vi "hostCommander_dualVStim_beta.vi"() -> ()   [LabVIEW 2014]
uses:
  <vilib>/Platform/TimedLoop/XDataNode/timing_clust.ctl
  <vilib>/Platform/TimedLoop/XDataNode/nitl_modes.ctl
  <vilib>/Platform/TimedLoop/XDataNode/wakeup.ctl
  <vilib>/dex/Stream Element Allocation Mode.ctl
  <vilib>/platform/TimedLoop/XDataNode/XDataNode.xnode
  <resource>/objmgr/ni.dex.rc
  <vilib>/Platform/TimedLoop/XDataNode/XDNodeRunTimeDep.lvlib
  <vilib>/Analysis/NI_AALBase.lvlib
  <vilib>/Analysis/1siggen.llb/Riffle Array (I32).vi
panel:
  in  "allowCorrection 2":bool
  out "Tab Control":enum32{"Host Commander"}(tab)
  out "rightReward":dbl format="%.2f"
  out "leftReward":dbl format="%.2f"
  out "rightLick":dbl format="%.2f"
  out "leftLick":dbl format="%.2f"
  out "reward#":i32=500
  in  "tickRate":u32=1
  in  "displayLength":dbl=10.0
  out "CurTrial#":u16
  out "Digital Waveform Graph":digitalwaveform(graph)
  out "stateMissed":bool
  out "VSmissed":bool
  out "VSbusy":bool=TRUE caption="VS"
  out "stateBusy":bool=TRUE caption="State"
  in  "FileName":string="debug"
  in  "Save data":bool=TRUE
  in  "Tab Control _2":T1(tab)
  in  "trialKey":i32[](array[numeric])
  in  "left":dbl=0.5 format="%.2f"
  in  "right":dbl=0.5 format="%.2f"
  in  "Initializeation Screen":dbl
  in  "Repeat":dbl
  in  "Interleave":bool
  in  "Randominze":bool
  in  "Blank":bool
  in  "Timing":sgl[](array[numeric])=[0.1, 0.2, 0.4, 0.6, 0.8, 1.0]
  in  "Orientation":sgl[](array[numeric])=[0.1, 0.2, 0.4, 0.6, 0.8, 1.0]
  in  "TF":sgl[](array[numeric])=[0.1, 0.2, 0.4, 0.6, 0.8, 1.0]
  in  "VS type":string(combo)="DelayedMatchToSampleMove"
  in  "SF":sgl[](array[numeric])=[0.04, 0.08, 0.16, 0.32, 0.45]
  in  "rtFIFOsize":u32=50
  in  "rtFIFOtimeout":u32
  in  "rtFIFOdataPool":u32=20
  in  "stateMachineCycle_uS":i64=500
  in  "minDelay":i32
  in  "maxDelay":i32=2000000
  in  "autoAllowCorrection":bool=TRUE
  in  "allowCorrection":bool
  in  "autoDelay":bool
  in  "vsFilterPeriod_uS":i32=500 format="%#1.6f"
  in  "lickThreshold_V":fxp<+/-,16,5>=1.0 format="%#.4f"
  in  "vsThreshold_V":fxp<+/-,16,5>=2.0 format="%#.4f"
  in  "audioThreshold_V":fxp<+/-,16,5>=2.2998046875 format="%.4f"
  in  "audioFilterPeriod_uS":i32=500 format="%#1.6f"
  in  "audioOffState_V":fxp<+/-,16,5> format="%#.4f"
  in  "manualShock":bool
  in  "manualWaterRight":bool
  in  "manualWaterLeft":bool
  in  "lickReward":bool
  in  "allowPunish":bool
  in  "beh type":string="LeftRight"
  in  "toneReward":bool
  in  "rwdrefPeriod_uS":u32=1000000
  in  "rewardPeriod_uS":u32=3000000
  in  "waterOn_uS":u32=35000
  in  "timeout_uS":u32=5000000
  in  "shockOn_uS":u32
  in  "delay_uS":u32=500000
  out "current state":u16(ring) items=["idle", "vs before", "vs", "vs after", "delay", "tone before", "tone", "tone after", "cycle end", "reward", "reward refractory", "punish", "punish refractory", "timeout", "exit"]
  out "case2":i32
  out "case1":i32
  in  "forceLeftTrial":bool
  in  "forceRightTrial":bool
  in  "forceCorrTrial":bool
  in  "autoCorrTrial":bool=TRUE
  in  "autoTimeout":bool
  in  "autoStop":bool
  in  "autoStopAtReward#":i32=250
  in  "updateEveryTrial#":u16=10
  in  "maxTimeout":i32=8000000
  out "newStartTrial#":i32
  out "newStartReward#":i32
  out "contNoRewardAccum":i32
  out "contNoReward":i32
  out "contReward":i32
  out "curPerformance":dbl format="%.2f"
  out "overallPerformance":dbl format="%.2f"
  in  "waterPunish":bool
  in  "No VS":bool
  out "Error 1":string
  out "Error 2":string
  out "Originating IP":string="192.168.137.2"
  out "Incoming data":string="TrlDone 1.000 "
  out "stream counter":u32
  out "Is Connected":bool
  out "Available Elements for Writing":i32
  in  "stream writer buffer size":i32=500
  in  "IP_VS":string="192.168.137.3"
  in  "IP_RT":string="192.168.137.2"
  in  "port_remote":u16=9091
  in  "IP_host":string="192.168.137.1"
  in  "port_local":u16=9090
  in  "IP_broadcast":string="192.168.137.255"
  out "INFO":string="Stop 1.000 "
  out "stop - local":bool=TRUE
  in  "Notes":string="14-4"
  in  "Abort":bool caption="run-stop"
  in  "run-stop":bool
  out "dispTimeout":bool
  out "saveTimeout":bool
  out "CurTrial# (remote)":u16
  in  "totalTrial#":u16=600
  out "CurTime":i32
  in  "ITI_ms":dbl=2000.0
  out "CurTime (sec)":i32
  in  "FilePath":string="D:\\BehData\\"
  # "busy"
  # "missed"
  # "min"
  # "sec"
  # "trialProbability"
  # "Errors for debugging"
types:
  T1 = enum32{"Visual Stimuli", "State Machine", "Behavior", "Network", "Notes"}
  T2 = enum16{"open", "replace", "create", "open or create", "replace or create", "replace or create with confirmation"}
  T3 = enum16{"big-endian, network order", "native, host order", "little-endian"}
  T4 = typedef "XDNodeRunTimeDep.lvlib/timing_clust.ctl" = cluster{"Expected End [f-1]":u64, "Actual End [f-1]":u64, "Finished Late? [f-1]":bool, "Expected End [i-1]":u64, "Actual End [i-1]":u64, "Finished Late? [i-1]":bool, "Expected Start [i]":u64, "Actual Start [i]":u64, "Expected Start [f]":u64, "Actual Start [f]":u64, "Source Name":string, "Structure Name":string, "Period":i64, "Deadline":i64, "Offset":i64, "Start":i64, "Priority":i32, "Timeout":i32, "Mode":T5, "Wakeup Reason":T6, "Error":errorcluster, "Source Type":string, "Secondary Source Type":string, "Global End Time":u64, "Global Start Time":u64, "Frame Duration":u64, "Iteration Duration":u64, "Assigned CPU":i32, "I/O Scan Engine Mode":u32}
  T5 = typedef "XDNodeRunTimeDep.lvlib/nitl_modes.ctl" = enum32{"No Change", "Process missed periods, maintain original phase", "Discard missed periods, maintain original phase", "Process missed periods, ignore original phase", "Discard missed periods, ignore original phase"}
  T6 = typedef "XDNodeRunTimeDep.lvlib/wakeup.ctl" = enum32{"Normal", "Aborted", "Asynchronous wakeup", "Timing source error", "Timed loop error", "Timeout"}
  T7 = typedef "Stream Element Allocation Mode.ctl" = u32
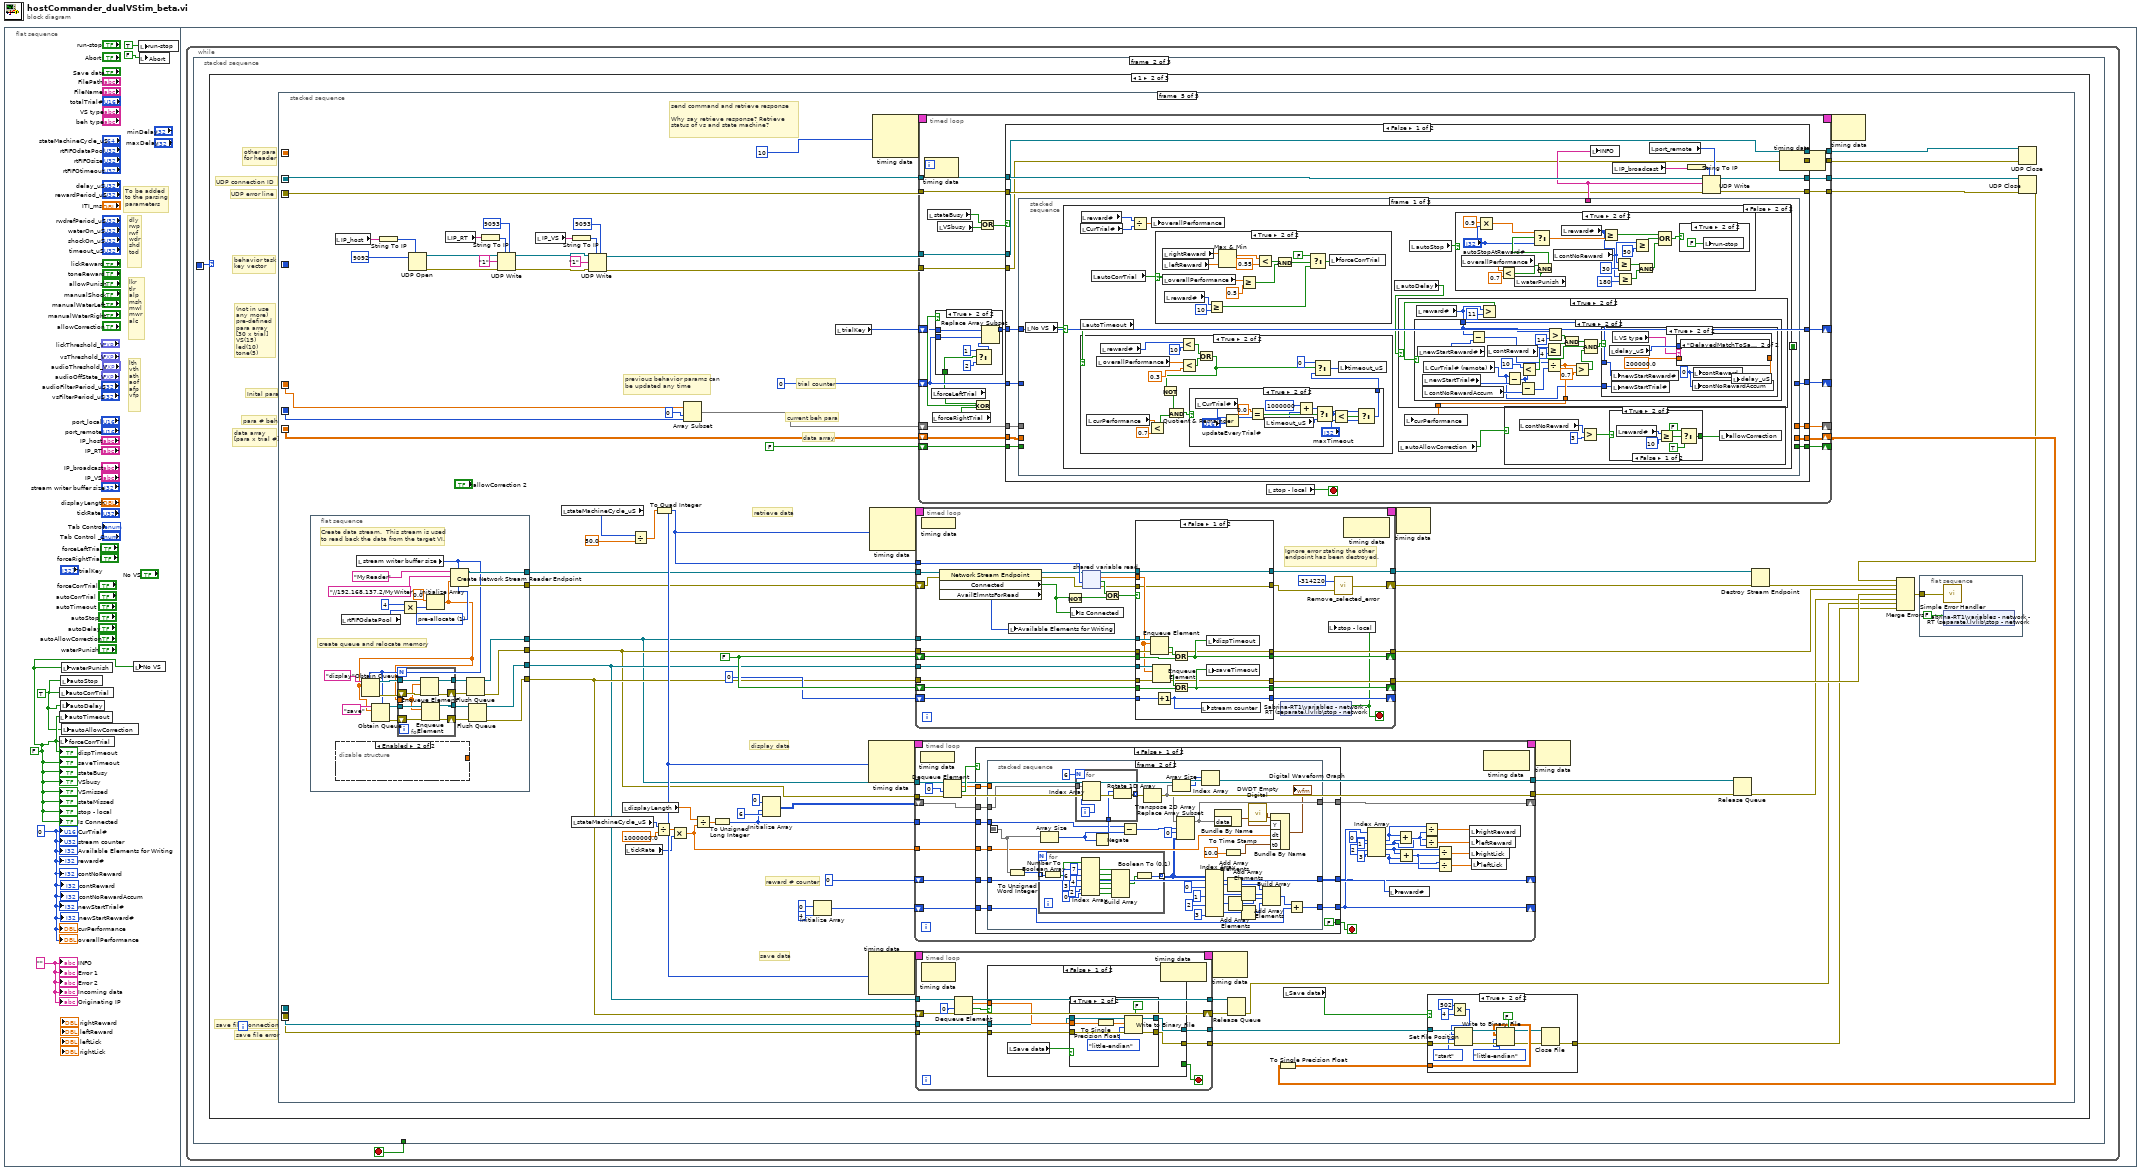
[diagram p0: block diagram]
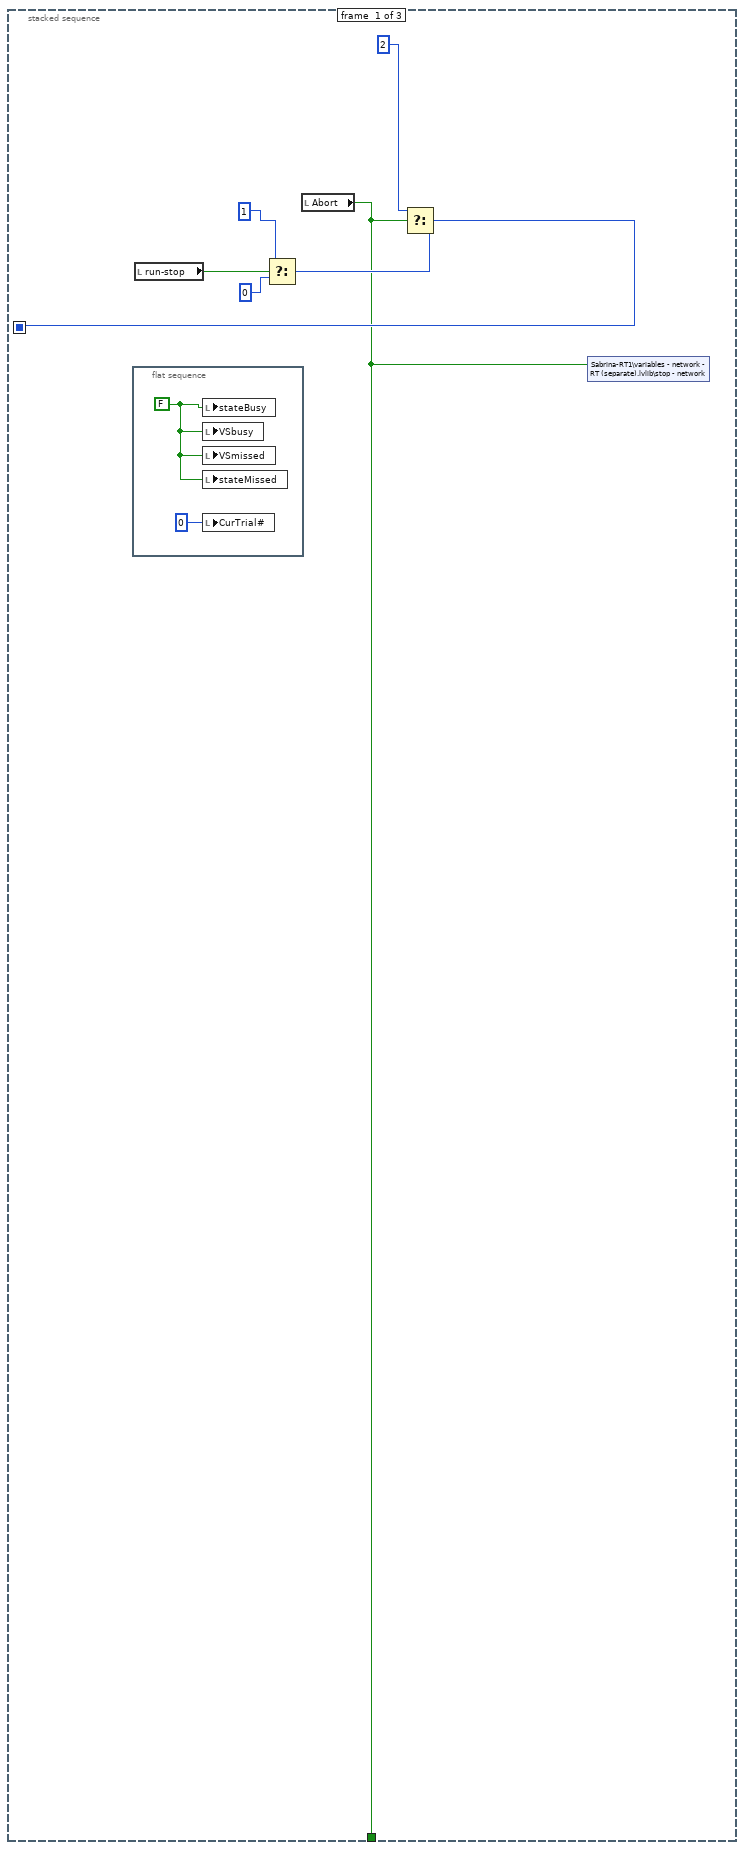
[diagram p2: hidden frame]
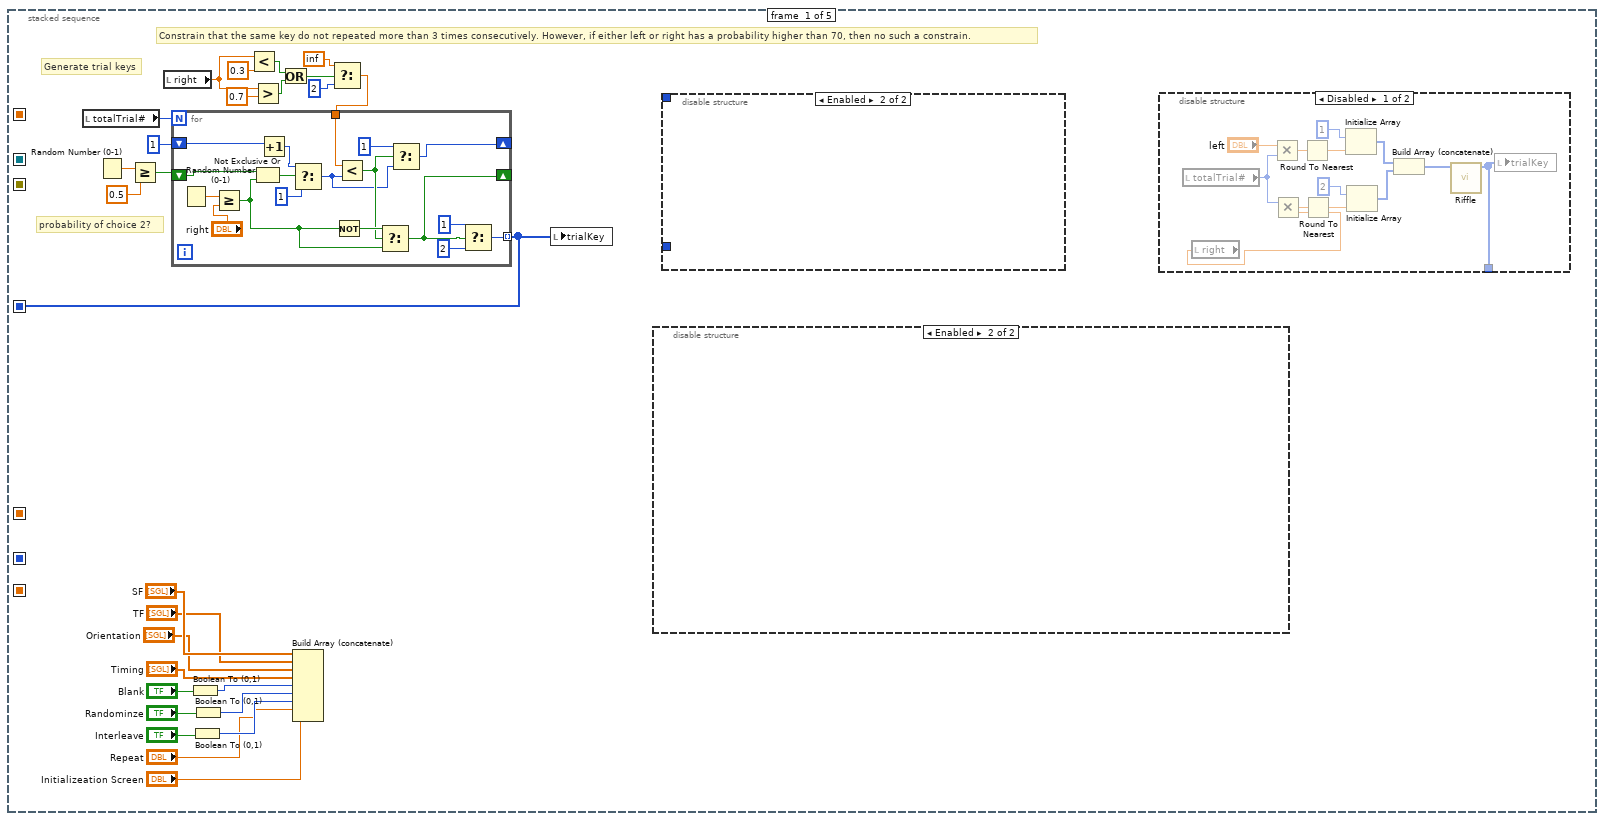
[diagram p4: hidden frame]
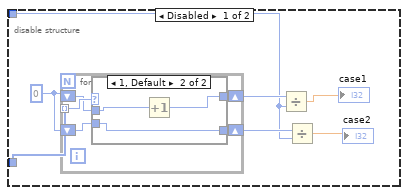
[diagram p5: hidden frame]
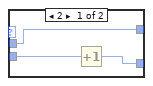
[diagram p6: hidden frame]
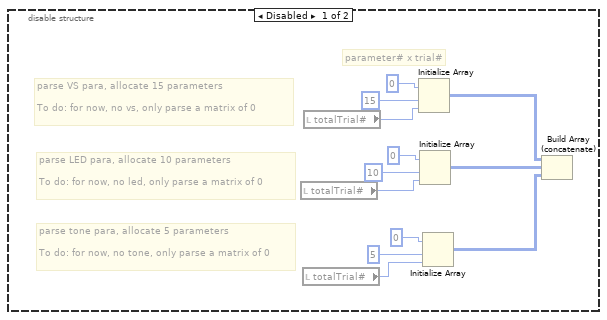
[diagram p8: hidden frame]
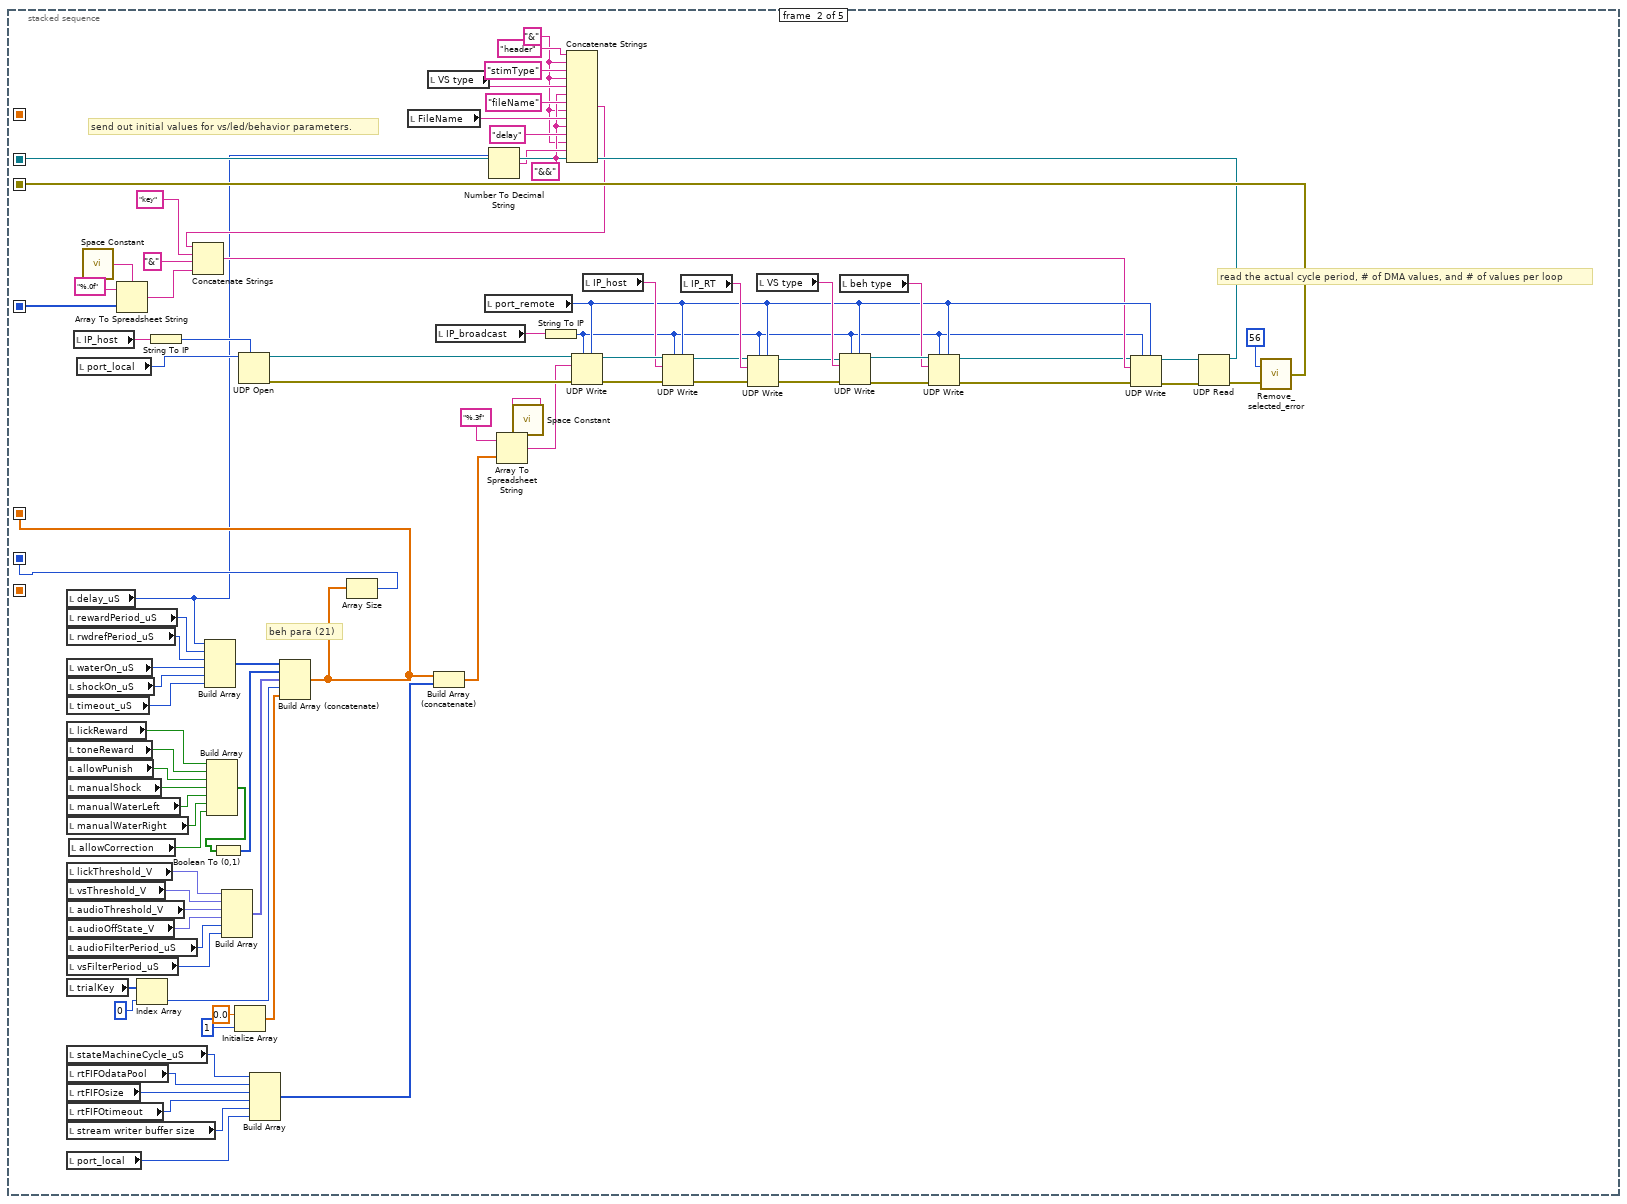
[diagram p9: hidden frame]
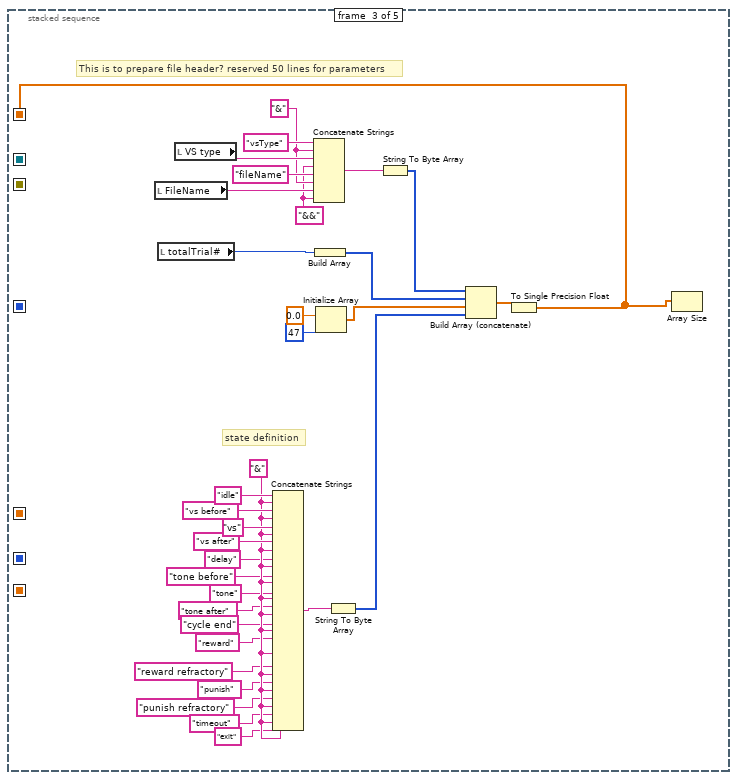
[diagram p10: hidden frame]
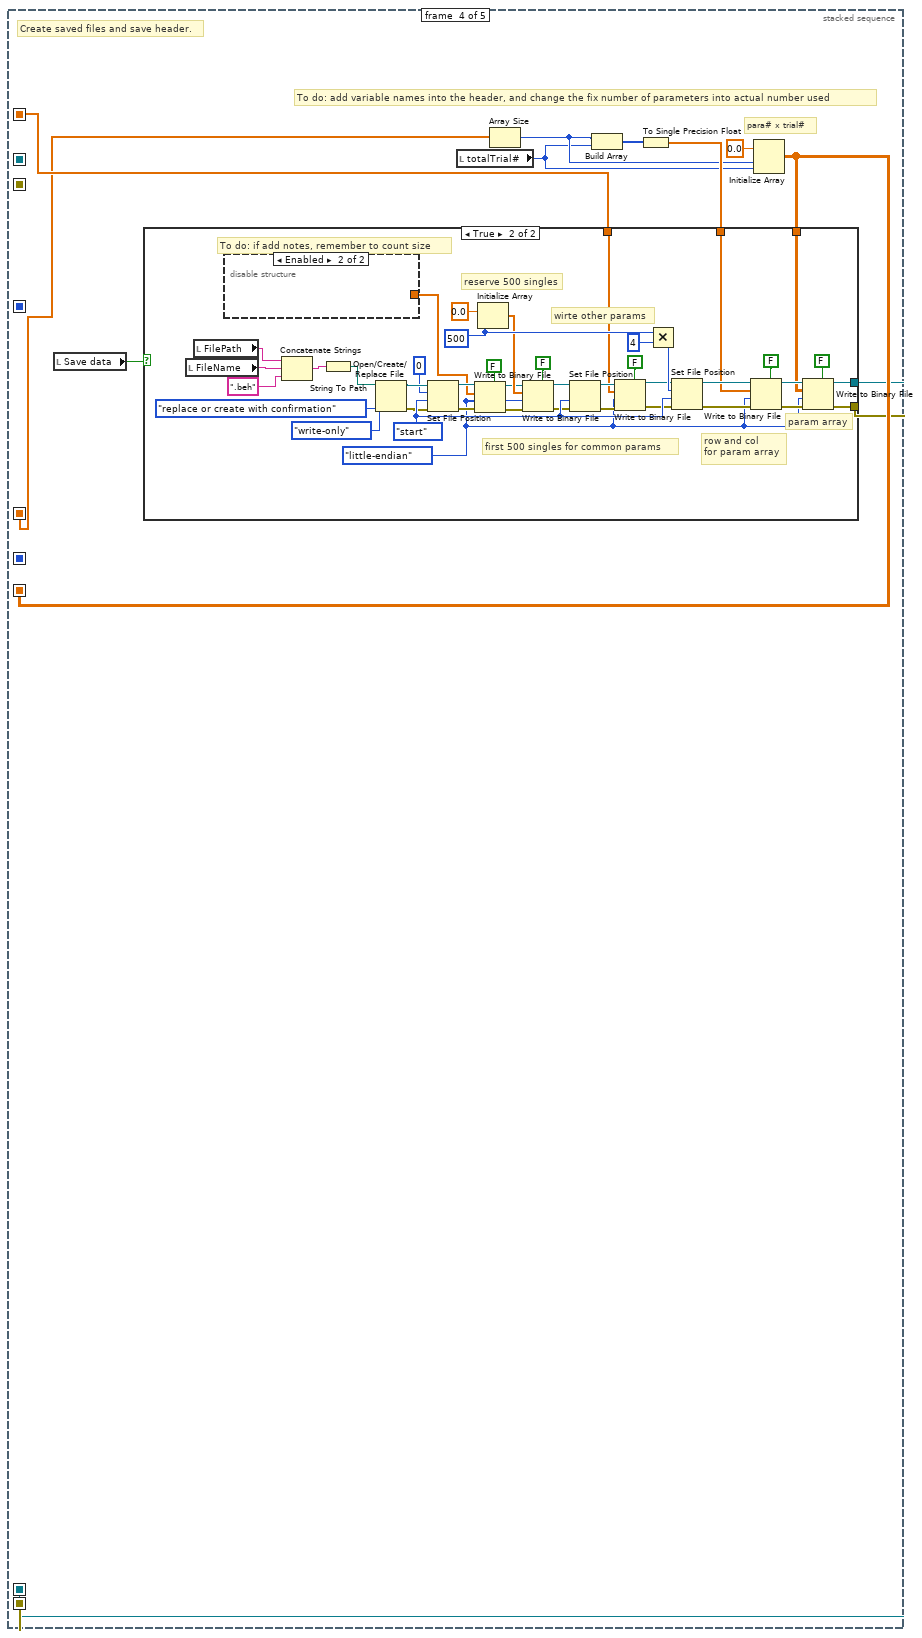
[diagram p11: hidden frame]
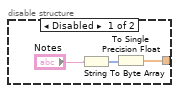
[diagram p13: hidden frame]
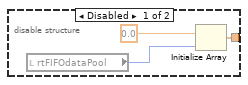
[diagram p14: hidden frame]
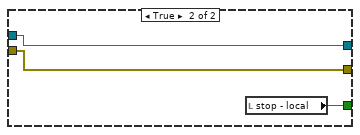
[diagram p16: hidden frame]
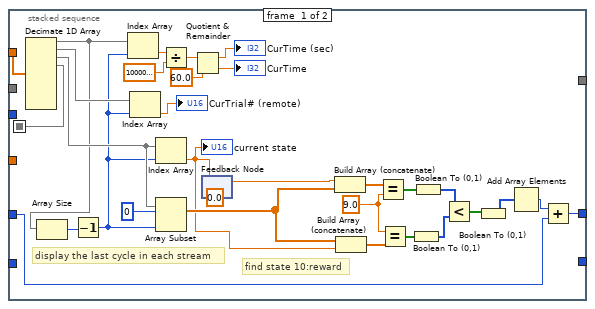
[diagram p17: hidden frame]
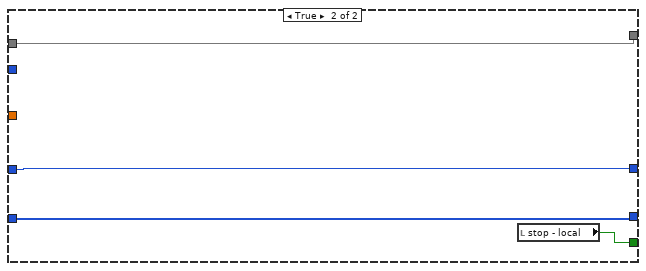
[diagram p18: hidden frame]
diagram:
  n1 = flat-sequence {
    frame #0 {
      w1 = TRUE
      w4 = ""
      w3 = 0
      w2 = FALSE
      # "To be added\nto the parsing\nparameters"
      # "lth\nvth\nath\naof\nafp\nvfp"
      # "dly\nrwp\nrwf\nwdr\nshd\ntod"
      # "lkr\ntlr\nalp\nmsh\nmwl\nmwr\nalc"
      n2 = local write "autoTimeout"(w2) -> ()
      n3 = local write "forceCorrTrial"(w2) -> ()
      n4 = local write "autoCorrTrial"(w1) -> ()
      n5 = local write "autoDelay"(w1) -> ()
      n6 = local write "autoStop"(w1) -> ()
      n7 = local write "waterPunish"(w2) -> ()
      n8 = local write "autoAllowCorrection"(w1) -> ()
      n9 = local write "No VS"(w2) -> ()
      n10 = local write "run-stop"(TRUE) -> ()
      n11 = local write "Abort"(FALSE) -> ()
      "dispTimeout" <- w2
      "saveTimeout" <- w2
      "stateBusy" <- w2
      "VSbusy" <- w2
      "VSmissed" <- w2
      "stateMissed" <- w2
      "CurTrial#" <- w3
      "stop - local" <- w2
      "INFO" <- w4
      "Error 2" <- w4
      "Error 1" <- w4
      "Available Elements for Writing" <- w3
      "Is Connected" <- w2
      "stream counter" <- w3
      "Incoming data" <- w4
      "Originating IP" <- w4
      "reward#" <- w3
      "contNoReward" <- w3
      "contReward" <- w3
      "contNoRewardAccum" <- w3
      "newStartTrial#" <- w3
      "newStartReward#" <- w3
      "curPerformance" <- w3
      "overallPerformance" <- w3
    }
    frame #1 {
      n12 = while {
        stop <- w7 stop-if-true
        n13 = stacked-sequence {
          seq-local: [w9 _ _] -> [_ w17 _]
          tunnel: [w8 _ _] -> w7
          frame #0 {
            n14 = flat-sequence {
              frame #0 {
                w16 = FALSE
                n15 = local write "stateBusy"(w16) -> ()
                n16 = local write "VSbusy"(w16) -> ()
                n17 = local write "VSmissed"(w16) -> ()
                n18 = local write "stateMissed"(w16) -> ()
                n19 = local write "CurTrial#"(0) -> ()
              }
            }
            n20 = local read "run-stop"() -> (w11:bool)
            n21 = Select(t=u8 1, s=w11, f=u8 0) -> (s? t:f=w10:u8)
            n22 = local read "Abort"() -> (w8:bool)
            n23 = Select(t=u8 2, s=w8, f=w10) -> (s? t:f=w9:u8)
            n24 = shared-variable "Sabrina-RT1\\variables - network - RT (separate).lvlib\\stop - network"(w8) -> ()  [unwired: 1 in, 1 out]
          }
          frame #1 {
            n25 = case shown="1" w17 {
              frame 0, Default {
              }
              frame 1 {
                # "behavior task\nkey vector"
                # "para # beh"
                # "save file error"
                # "save file connection"
                # "data array\n[para x trial #]"
                # "other para\nfor header"
                # "UDP error line"
                # "UDP connection ID"
                # "Inital para"
                # "(not in use any more) pre-defined \npara array\n[30 x trial]\nVS(15)\nled(10)\ntone(5)"
                n26 = stacked-sequence {
                  seq-local: [_ w176 _ _ _] -> [_ _ _ _ w355]
                  seq-local: [_ w175 _ _ _] -> [_ _ _ _ w356]
                  seq-local: [_ w136 _ _ _] -> [_ _ _ w228 w304]
                  seq-local: [w18 _ _ _ _] -> [_ w132 _ _ _]
                  seq-local: [_ _ w196 _ _] -> [_ _ _ w232 _]
                  seq-local: [_ _ _ w231 _] -> [_ _ _ _ w349]
                  seq-local: [_ _ _ w230 _] -> [_ _ _ _ w329]
                  seq-local: [_ _ _ w229 _] -> [_ _ _ _ w330]
                  seq-local: [_ w145 _ _ _] -> [_ _ _ _ w310]
                  frame #0 {
                    # "probability of choice 2?"
                    # "Constrain that the same key do not repeated more than 3 times consecutively. However, if either left or right has a probability higher than 70, then no such a constrain."
                    # "Generate trial keys"
                    n27 = local read "totalTrial#"() -> (w19:u16)
                    n28 = Random Number (0-1)() -> (number: 0 to 1=w32:dbl)
                    n29 = Greater Or Equal?(x=w32, y=0.5) -> (x >= y?=w30:bool)
                    n30 = local read "right"() -> (w26:dbl)
                    n31 = Boolean To (0,1)(Boolean="Blank") -> (0, 1=w39:i16)
                    n32 = Boolean To (0,1)(Boolean="Interleave") -> (0, 1=w34:i16)
                    n33 = Boolean To (0,1)(Boolean="Randominze") -> (0, 1=w38:i16)
                    n34 = Less?(x=w26, y=0.3) -> (x < y?=w23:bool)
                    n35 = Greater?(x=w26, y=0.7) -> (0:w22:bool)
                    n36 = Or(x=w23, y=w22) -> (x .or. y?=w21:bool)
                    n37 = Build Array (concatenate)("SF", "TF", "Orientation", "Timing", w39, w38, w34, "Repeat", "Initializeation Screen") -> ()  [unwired: 1 out]
                    n38 = Select(t=inf, s=w21, f=2) -> (s? t:f=w20:dbl)
                    n39 = for {
                      N: w19 -> [_]
                      shift-right: [w79] -> _
                      shift-left: w30 -> [w92]
                      shift-right: [w77] -> _
                      shift-left: 1 -> [w90]
                      tunnel: w20 -> [w80]
                      tunnel: [w78] -> w18 mode=indexing
                      n40 = Random Number (0-1)() -> (number: 0 to 1=w93:dbl)
                      n41 = Greater Or Equal?(x=w93, y="right") -> (x >= y?=w83:bool)
                      n42 = Not Exclusive Or(1:w83, 2:w92) -> (0:w91:bool)
                      n43 = Increment(x=w90) -> (x+1=w87:i32)
                      n44 = Select(t=w87, s=w91, f=1) -> (s? t:f=w81:i32)
                      n45 = Not(x=w83) -> (.not. x?=w84:bool)
                      n46 = Less?(x=w80, y=w81) -> (x < y?=w82:bool)
                      n47 = Select(t=w84, s=w82, f=w83) -> (s? t:f=w79:bool)
                      n48 = Select(t=1, s=w82, f=w81) -> (s? t:f=w77:i32)
                      n49 = Select(t=1, s=w79, f=2) -> (s? t:f=w78:i32)
                    }
                    n50 = local write "trialKey"(w18) -> ()
                    n51 = disable-structure shown="Enabled" {
                      frame Disabled {
                        # "parameter# x trial#"
                        # "parse tone para, allocate 5 parameters \n\nTo do: for now, no tone, only parse a matrix of 0"
                        # "parse LED para, allocate 10 parameters \n\nTo do: for now, no led, only parse a matrix of 0"
                        # "parse VS para, allocate 15 parameters \n\nTo do: for now, no vs, only parse a matrix of 0"
                        n52 = local read "totalTrial#"() -> (w99:u16)
                        n53 = local read "totalTrial#"() -> (w98:u16)
                        n54 = local read "totalTrial#"() -> (w100:u16)
                        n55 = Initialize Array(0, 15, w100) -> (w103:i32[][])
                        n56 = Initialize Array(0, 10, w99) -> (w102:i32[][])
                        n57 = Initialize Array(0, 5, w98) -> (w101:i32[][])
                        n58 = Build Array (concatenate)(w103, w102, w101) -> ()  [unwired: 1 out]
                      }
                      frame Enabled {
                      }
                    }
                    n59 = disable-structure shown="Enabled" {
                      disable-tunnel: _ -> [w51 _]
                      disable-tunnel: _ -> [w45 _]
                      frame Disabled {
                        w50 = 0
                        n60 = for {
                          tunnel: w51 -> [w56] mode=indexing
                          shift-right: [w54] -> w47
                          shift-left: w50 -> [w55]
                          shift-right: [w52] -> w49
                          shift-left: w50 -> [w53]
                          n61 = case shown="1, Default" w56 {
                            tunnel: w55 -> [w59 w60]
                            tunnel: [w58 w60] -> w54
                            tunnel: w53 -> [w57 w62]
                            tunnel: [w57 w61] -> w52
                            frame 2 {
                              n62 = Increment(x=w59) -> (x+1=w58:i32)
                            }
                            frame 1, Default {
                              n63 = Increment(x=w62) -> (x+1=w61:i32)
                            }
                          }
                        }
                        n64 = Divide(x=w49, y=w45) -> (x/y=→"case1":dbl)
                        n65 = Divide(x=w47, y=w45) -> (x/y=→"case2":dbl)
                      }
                      frame Enabled {
                      }
                    }
                    n66 = disable-structure shown="Disabled" {
                      disable-tunnel: [w64 _] -> _
                      frame Disabled {
                        n67 = local read "totalTrial#"() -> (w68:u16)
                        n68 = local read "right"() -> (w63:dbl)
                        n69 = Multiply(x="left", y=w68) -> (x*y=w74:dbl)
                        n70 = Multiply(x=w68, y=w63) -> (x*y=w69:dbl)
                        n71 = Round To Nearest(number=w74) -> (nearest integer value=w72:dbl)
                        n72 = Round To Nearest(number=w69) -> (nearest integer value=w71:dbl)
                        n73 = Initialize Array(1, w72) -> (w67:i32[])
                        n74 = Initialize Array(2, w71) -> (w66:i32[])
                        n75 = Build Array (concatenate)(w67, w66) -> (w65:i32[])
                        n76 = call-poly <vilib>:"Riffle.vi"("X"=w65) -> ("Riffled {X}"=w64:i32[])  [unwired: 8 in, 2 out]
                        n77 = local write "trialKey"(w64) -> ()
                      }
                      frame Enabled {
                      }
                    }
                  }
                  frame #1 {
                    w106 = "&" ("string")
                    w108 = "&&" ("string")
                    # "beh para (21)"
                    # "read the actual cycle period, # of DMA values, and # of values per loop"
                    # "send out initial values for vs/led/behavior parameters."
                    n78 = local read "delay_uS"() -> (w110:u32)
                    n79 = local read "rewardPeriod_uS"() -> (w172:u32)
                    n80 = local read "rwdrefPeriod_uS"() -> (w171:u32)
                    n81 = local read "waterOn_uS"() -> (w170:u32)
                    n82 = local read "shockOn_uS"() -> (w169:u32)
                    n83 = local read "timeout_uS"() -> (w168:u32)
                    n84 = local read "lickReward"() -> (w167:bool)
                    n85 = local read "toneReward"() -> (w166:bool)
                    n86 = local read "allowPunish"() -> (w165:bool)
                    n87 = local read "manualShock"() -> (w164:bool)
                    n88 = local read "manualWaterLeft"() -> (w163:bool)
                    n89 = local read "manualWaterRight"() -> (w162:bool)
                    n90 = local read "lickThreshold_V"() -> (w161:fxp<+/-,16,5>)
                    n91 = local read "vsThreshold_V"() -> (w160:fxp<+/-,16,5>)
                    n92 = local read "audioThreshold_V"() -> (w159:fxp<+/-,16,5>)
                    n93 = local read "audioOffState_V"() -> (w156:fxp<+/-,16,5>)
                    n94 = local read "audioFilterPeriod_uS"() -> (w158:i32)
                    n95 = local read "vsFilterPeriod_uS"() -> (w157:i32)
                    n96 = local read "trialKey"() -> (w121:i32[])
                    n97 = local read "stateMachineCycle_uS"() -> (w155:i64)
                    n98 = local read "rtFIFOdataPool"() -> (w153:u32)
                    n99 = local read "rtFIFOsize"() -> (w152:u32)
                    n100 = local read "rtFIFOtimeout"() -> (w154:u32)
                    n101 = local read "stream writer buffer size"() -> (w151:i32)
                    n102 = local read "port_local"() -> (w144:u16)
                    n103 = local read "allowCorrection"() -> (w117:bool)
                    n104 = local read "IP_host"() -> (w189:string)
                    n105 = local read "port_local"() -> (w188:u16)
                    n106 = call <vilib>:"Space Constant.vi"() -> ("String"=w126:string)
                    n107 = Array To Spreadsheet String ("beh para")(delimiter (Tab)=w126, array=w132, 3:"%.0f" ("format string")) -> (spreadsheet string=w128:string)
                    n108 = Index Array(array=w121, index=0) -> (element=w118:i32)
                    n109 = String To IP(1:w189) -> (0:w122:u32)
                    n110 = Build Array(w110, w172, w171, w170, w169, w168) -> (w150:u32[])
                    n111 = Build Array(w167, w166, w165, w164, w163, w162, w117) -> (w138:bool[])
                    n112 = Boolean To (0,1)(Boolean=w138) -> (0, 1=w137:i16[])
                    n113 = Build Array(w161, w160, w159, w156, w158, w157) -> (w149:fxp<+/-,43,32>[])
                    n114 = Initialize Array(sgl 0.0, 1) -> (w119:sgl[])
                    n115 = UDP Open(7:w122, 11:w188) -> (port=w186:refnum<k16>, 0:w187:errorcluster)  [unwired: 3 in, 1 out]
                    n116 = Build Array(w155, w153, w152, w154, w151, w144) -> (w148:i64[])
                    n117 = Build Array (concatenate)(w150, w137, w149, w118, w119) -> (w136:sgl[])
                    n118 = Array Size(array=w136) -> (size(s)=w145:i32)
                    n119 = local read "FileName"() -> (w116:string)
                    n120 = local read "VS type"() -> (w113:string)
                    n121 = Build Array (concatenate)(w136, w148) -> (w177:sgl[])
                    n122 = local read "IP_broadcast"() -> (w190:string)
                    n123 = local read "port_remote"() -> (w129:u16)
                    n124 = Number To Decimal String(number=w110) -> (decimal integer string=w109:string)  [unwired: 1 in]
                    n125 = call <vilib>:"Space Constant.vi"() -> ("String"=w179:string)
                    n126 = Array To Spreadsheet String ("beh para")(delimiter (Tab)=w179, array=w177, 3:"%.3f" ("format string")) -> (spreadsheet string=w178:string)
                    n127 = String To IP(1:w190) -> (0:w123:u32)
                    n128 = Concatenate Strings("header" ("string"), w106, "stimType" ("string"), w106, w113, w108, "fileName" ("string"), w106, w116, w108, "delay" ("string"), w106, w109, w108) -> (w112:string)
                    n129 = Concatenate Strings(w112, "key", "&", w128) -> (w127:string)
                    n130 = UDP Write(address=w123, port or service name=w129, connection ID=w186, data in=w178, 8:w187) -> (error out=w185:errorcluster, 3:w143:refnum<k16>)  [unwired: 1 in]
                    n131 = local read "IP_host"() -> (w142:string)
                    n132 = UDP Write(address=w123, port or service name=w129, connection ID=w143, data in=w142) -> (3:w140:refnum<k16>)  [unwired: 2 in, 1 out]
                    n133 = local read "IP_RT"() -> (w141:string)
                    n134 = UDP Write(address=w123, port or service name=w129, connection ID=w140, data in=w141) -> (3:w139:refnum<k16>)  [unwired: 2 in, 1 out]
                    n135 = local read "VS type"() -> (w184:string)
                    n136 = local read "beh type"() -> (w181:string)
                    n137 = UDP Write(address=w123, port or service name=w129, connection ID=w139, data in=w184, 8:w185) -> (error out=w183:errorcluster, 3:w182:refnum<k16>)  [unwired: 1 in]
                    n138 = UDP Write(address=w123, port or service name=w129, connection ID=w182, data in=w181, 8:w183) -> (error out=w124:errorcluster, 3:w125:refnum<k16>)  [unwired: 1 in]
                    n139 = UDP Write(address=w123, port or service name=w129, connection ID=w125, data in=w127, 8:w124) -> (error out=w135:errorcluster, 3:w134:refnum<k16>)  [unwired: 1 in]
                    n140 = UDP Read(connection ID=w134, 8:w135) -> (error out=w174:errorcluster, 3:w175:refnum<k16>)  [unwired: 2 in, 3 out]
                    n141 = call "Remove_selected_error.vi"("error in (no error)"=w174, "errorCode"=56) -> ("error out"=w176:errorcluster)
                  }
                  frame #2 {
                    w193 = "&" ("string")
                    w191 = "&&" ("string")
                    w208 = "&" ("string")
                    # "state definition"
                    # "This is to prepare file header? reserved 50 lines for parameters"
                    n142 = local read "FileName"() -> (w192:string)
                    n143 = local read "totalTrial#"() -> (w216:u16)
                    n144 = local read "VS type"() -> (w211:string)
                    n145 = Concatenate Strings("idle", w208, "vs before", w208, "vs", w208, "vs after", w208, "delay", w208, "tone before", w208, "tone", w208, "tone after", w208, "cycle end", w208, "reward", w208, "reward refractory", w208, "punish", w208, "punish refractory", w208, "timeout", w208, "exit", w208) -> (w221:string)
                    n146 = Concatenate Strings("vsType" ("string"), w193, w211, w191, "fileName" ("string"), w193, w192, w191) -> (w210:string)
                    n147 = Build Array(w216) -> (w215:u16[])
                    n148 = Initialize Array(sgl 0.0 ("element"), 47 ("dimension size")) -> (w214:sgl[])
                    n149 = String To Byte Array(string=w221) -> (unsigned byte array=w213:u8[])
                    n150 = String To Byte Array(string=w210) -> (unsigned byte array=w209:u8[])
                    n151 = Build Array (concatenate)(w209, w215, w214, w213) -> (w212:sgl[])
                    n152 = To Single Precision Float(number=w212) -> (single precision float=w196:sgl[])
                    n153 = Array Size(array=w196) -> ()  [unwired: 1 out]
                  }
                  frame #3 {
                    # "To do: add variable names into the header, and change the fix number of parameters into actual number used"
                    # "para# x trial#"
                    # "Create saved files and save header."
                    n154 = local read "Save data"() -> (w234:bool)
                    n155 = local read "totalTrial#"() -> (w224:u16)
                    n156 = Array Size(array=w228) -> (size(s)=w225:i32)
                    n157 = Build Array(w225, w224) -> (w227:i32[])
                    n158 = To Single Precision Float(number=w227) -> (single precision float=w226:sgl[])
                    n159 = Initialize Array(sgl 0.0 ("element"), w225, w224) -> (w231:sgl[][])
                    n160 = case shown="True" w234 {
                      tunnel: w226 -> [_ w251]
                      tunnel: w232 -> [_ w235]
                      tunnel: w231 -> [_ w250]
                      tunnel: [_ w248] -> w229
                      tunnel: [_ w249] -> w230
                      frame False {
                      }
                      frame True {
                        w269 = 500 ("dimension size")
                        w242 = T3."little-endian" ("byte order (0:big-endian, network order)")
                        w270 = enum16{"start", "end", "current"}."start" ("from (0:start)")
                        # "To do: if add notes, remember to count size"
                        # "param array"
                        # "row and col\nfor param array"
                        # "first 500 singles for common params"
                        # "reserve 500 singles"
                        # "wirte other params"
                        n161 = local read "FileName"() -> (w237:string)
                        n162 = local read "FilePath"() -> (w240:string)
                        n163 = disable-structure shown="Enabled" {
                          disable-tunnel: [w277 _] -> w241
                          frame Disabled {
                            n164 = String To Byte Array(string="Notes") -> (unsigned byte array=w278:u8[])
                            n165 = To Single Precision Float(number=w278) -> (single precision float=w277:sgl[])
                          }
                          frame Enabled {
                          }
                        }
                        n166 = Concatenate Strings(w240, w237, ".beh" ("string")) -> (w239:string)
                        n167 = String To Path(string=w239) -> (path=w238:path)
                        n168 = Open/Create/Replace File(file path (use dialog)=w238, operation (0:open)=T2."replace or create with confirmation", access (0:read/write)=enum16{"read/write", "read-only", "write-only"}."write-only") -> (refnum out=w255:refnum<file>, error out=w256:errorcluster)  [unwired: 3 in, 1 out]
                        n169 = Set File Position(offset (in bytes) (0)=i64 0, refnum=w255, from (0:start)=w270, error in=w256) -> (refnum out=w246:refnum<file>, error out=w244:errorcluster)
                        n170 = Write to Binary File(file (use dialog)=w246, data=w241, error in=w244, 5:FALSE ("prepend array or string size? (T)"), 9:w242) -> (refnum out=w245:refnum<file>, error out=w243:errorcluster)  [unwired: 1 in, 1 out]
                        n171 = Initialize Array(sgl 0.0 ("element"), w269) -> (w259:sgl[])
                        n172 = Write to Binary File(file (use dialog)=w245, data=w259, error in=w243, 5:FALSE ("prepend array or string size? (T)"), 9:w242) -> (refnum out=w261:refnum<file>, error out=w262:errorcluster)  [unwired: 1 in, 1 out]
                        n173 = Set File Position(refnum=w261, from (0:start)=w270, error in=w262) -> (refnum out=w263:refnum<file>, error out=w264:errorcluster)  [unwired: 1 in]
                        n174 = Write to Binary File(file (use dialog)=w263, data=w235, error in=w264, 5:FALSE ("prepend array or string size? (T)"), 9:w242) -> (refnum out=w265:refnum<file>, error out=w266:errorcluster)  [unwired: 1 in, 1 out]
                        n175 = Multiply(x=w269, y=4) -> (x*y=w267:i32)
                        n176 = Set File Position(offset (in bytes) (0)=w267, refnum=w265, from (0:start)=w270, error in=w266) -> (refnum out=w272:refnum<file>, error out=w273:errorcluster)
                        n177 = Write to Binary File(file (use dialog)=w272, data=w251, error in=w273, 5:FALSE ("prepend array or string size? (T)"), 9:w242) -> (refnum out=w274:refnum<file>, error out=w275:errorcluster)  [unwired: 1 in, 1 out]
                        n178 = Write to Binary File(file (use dialog)=w274, data=w250, error in=w275, 5:FALSE ("prepend array or string size? (T)"), 9:w242) -> (refnum out=w248:refnum<file>, error out=w249:errorcluster)  [unwired: 1 in, 1 out]
                      }
                    }
                  }
                  frame #4 {
                    w361 = FALSE
                    # "reward # counter"
                    # "save data"
                    # "data array"
                    # "current beh para"
                    # "trial counter"
                    # "previous behavior params can be updated any time"
                    # "display data"
                    # "retrieve data"
                    # "send command and retrieve response\n\nWhy say retrieve response? Retrieve\nstatus of vs and state machine?"
                    n179 = flat-sequence {
                      tunnel: [w388] -> w316
                      tunnel: [w387] -> w315
                      tunnel: [w376] -> w314
                      tunnel: [w375] -> w313
                      tunnel: [w374] -> w312
                      tunnel: [w373] -> w311
                      frame #0 {
                        w390 = T7 1 items=["allocate as needed", "pre-allocate"] ("element allocation mode")
                        # "create queue and relocate memory"
                        # "Create data stream.  This stream is used\nto read back the data from the target VI."
                        n180 = disable-structure shown="Enabled" {
                          disable-tunnel: [w393 _] -> _
                          frame Disabled {
                            n181 = local read "rtFIFOdataPool"() -> (w394:u32)
                            n182 = Initialize Array(sgl 0.0, w394) -> (w393:sgl[])
                          }
                          frame Enabled {
                          }
                        }
                        n183 = local read "rtFIFOdataPool"() -> (w369:u32)
                        n184 = local read "stream writer buffer size"() -> (w372:i32)
                        n185 = Multiply(x=4, y=w369) -> (x*y=w368:u32)
                        n186 = Initialize Array(sgl 0.0, w368) -> (w371:sgl[])
                        n187 = Obtain Queue(max queue size (-1, unlimited)=w372, name (unnamed)="display", element data type=w371) -> (queue out=w379:refnum<queue>, error out=w380:errorcluster)  [unwired: 2 in, 1 out]
                        n188 = Obtain Queue(max queue size (-1, unlimited)=w372, name (unnamed)="save", element data type=w371) -> (queue out=w381:refnum<queue>, error out=w382:errorcluster)  [unwired: 2 in, 1 out]
                        n189 = for {
                          N: w372 -> [_]
                          tunnel: w379 -> [w404]
                          tunnel: [w403] -> w385
                          shift-right: [w401] -> w386
                          shift-left: w380 -> [w402]
                          shift-right: [w397] -> w384
                          shift-left: w382 -> [w398]
                          tunnel: w381 -> [w400]
                          tunnel: [w399] -> w383
                          tunnel: w371 -> [w396]
                          n190 = Enqueue Element(queue=w404, element=w396, error in (no error)=w402) -> (queue out=w403:refnum<queue>, error out=w401:errorcluster)  [unwired: 1 in, 1 out]
                          n191 = Enqueue Element(queue=w400, element=w396, error in (no error)=w398) -> (queue out=w399:refnum<queue>, error out=w397:errorcluster)  [unwired: 1 in, 1 out]
                        }
                        n192 = Create Network Stream Reader Endpoint(6:w390, 7:w372, 9:w371, 10:"//192.168.137.2/MyWriter" ("reader name"), 11:"MyReader" ("reader name")) -> (0:w388:errorcluster, 3:w387:refnum<k21>)  [unwired: 2 in]
                        n193 = Flush Queue(queue=w385, error in (no error)=w386) -> (queue out=w373:refnum<queue>, error out=w374:errorcluster)  [unwired: 1 out]
                        n194 = Flush Queue(queue=w383, error in (no error)=w384) -> (queue out=w375:refnum<queue>, error out=w376:errorcluster)  [unwired: 1 out]
                      }
                    }
                    n195 = local read "IP_host"() -> (w299:string)
                    n196 = String To IP(1:w299) -> (0:w298:u32)
                    n197 = UDP Open(7:w298, 11:9092) -> (port=w293:refnum<k16>, 0:w294:errorcluster)  [unwired: 3 in, 1 out]
                    n198 = local read "IP_RT"() -> (w292:string)
                    n199 = String To IP(1:w292) -> (0:w291:u32)
                    n200 = UDP Write(address=w291, port or service name=u16 9093, connection ID=w293, data in="1", 8:w294) -> (error out=w283:errorcluster, 3:w284:refnum<k16>)  [unwired: 1 in]
                    n201 = local read "IP_VS"() -> (w285:string)
                    n202 = local read "stateMachineCycle_uS"() -> (w364:i64)
                    n203 = local read "stateMachineCycle_uS"() -> (w343:i64)
                    n204 = String To IP(1:w285) -> (0:w286:u32)
                    n205 = UDP Write(address=w286, port or service name=u16 9093, connection ID=w284, data in="1", 8:w283) -> (error out=w281:errorcluster, 3:w282:refnum<k16>)  [unwired: 1 in]
                    n206 = local read "displayLength"() -> (w337:dbl)
                    n207 = local read "tickRate"() -> (w308:u32)
                    n208 = Divide(x=w364, y=sgl 50.0) -> (x/y=w363:sgl)
                    n209 = To Quad Integer(1:w363) -> (0:w317:i64)
                    n210 = Divide(x=w343, y=1000000.0) -> (x/y=w309:dbl)
                    n211 = Multiply(x=w309, y=w308) -> (x*y=w307:dbl)
                    n212 = Array Subset(array=w304, index=0, length=w310) -> (w354:sgl[])
                    n213 = Divide(x=w337, y=w307) -> (x/y=w340:dbl)
                    n214 = To Unsigned Long Integer(number=w340) -> (unsigned 32bit integer=w338:u32)
                    n215 = Initialize Array(u8 0, w338, 6 ("dimension size")) -> (w339:u8[][])
                    n216 = Initialize Array(u32 0, u32 4) -> (w301:u32[])
                    n217 = local read "trialKey"() -> (w280:i32[])
                    n218 = node-c288(w317) -> (w336:T4)  [unwired: 2 in]
                    n219 = node-c288(w317) -> (w334:T4)  [unwired: 2 in]
                    n220 = node-c288(w317) -> (w367:T4)  [unwired: 2 in]
                    n221 = node-c288(10) -> (w358:T4)  [unwired: 2 in]
                    n222 = timed-loop {
                      tunnel: w311 -> [w473]
                      tunnel: w312 -> [w472]
                      shift-right: [w444] -> _
                      shift-left: u32 0 -> [w461]
                      shift-right: [w467] -> _
                      shift-left: w339 -> [w469]
                      tunnel: w338 -> [w468]
                      timing: w336 -> [_]
                      timing-out: [_] -> w335
                      tunnel: [w464] -> w326
                      tunnel: [w463] -> w325
                      tunnel: w307 -> [w462]
                      shift-right: [w455] -> _
                      shift-left: w301 -> [w460]
                      stop <- w466 stop-if-true
                      n223 = node-c288() -> ()  [unwired: 1 in]
                      n224 = Dequeue Element(queue=w473, timeout in ms (-1)=0, error in (no error)=w472) -> (queue out=w464:refnum<queue>, element=w470:sgl[], timed out?=w471:bool, error out=w463:errorcluster)
                      n225 = case shown="False" w471 {
                        tunnel: w470 -> [w485 _]
                        tunnel: w461 -> [w484 w574]
                        tunnel: [w483 w574] -> w444
                        tunnel: w469 -> [w482 w575]
                        tunnel: w468 -> [w481 _]
                        tunnel: [w480 w575] -> w467
                        tunnel: [FALSE w576] -> w466
                        tunnel: w462 -> [w478 _]
                        tunnel: w460 -> [w477 w573]
                        tunnel: [w476 w573] -> w455
                        frame False {
                          n226 = stacked-sequence {
                            seq-local: [w487 _] -> [_ w544]
                            tunnel: w485 -> [w516 _]
                            tunnel: w484 -> [w501 _]
                            tunnel: [w506 _] -> w483
                            tunnel: w482 -> [_ w543]
                            tunnel: w481 -> [_ w535]
                            tunnel: [_ w538] -> w480
                            tunnel: w478 -> [_ w536]
                            tunnel: w477 -> [_ w518]
                            tunnel: [_ w517] -> w476
                            frame #0 {
                              w495 = sgl 9.0
                              # "display the last cycle in each stream"
                              # "find state 10:reward"
                              n227 = Decimate 1D Array(w516) -> (w502:sgl[], w504:sgl[], w503:sgl[], w487:sgl[])  [unwired: 5 out]
                              n228 = Array Size(array=w502) -> (size(s)=w500:i32)
                              n229 = Decrement(x=w500) -> (x-1=w499:i32)
                              n230 = Index Array(array=w502, index=w499) -> (element=w507:sgl)
                              n231 = Index Array(array=w504, index=w499) -> (element=→"CurTrial# (remote)":sgl)
                              n232 = Index Array(array=w503, index=w499) -> (element=w497:sgl)
                              "current state" <- w497
                              n233 = Array Subset(array=w503, index=0, length=w499) -> (w498:sgl[])
                              n234 = Divide(x=w507, y=sgl 1000000.0) -> (x/y=w509:sgl)
                              n235 = Quotient & Remainder(x=w509, y=sgl 60.0) -> (x-y*floor(x/y)=→"CurTime (sec)":sgl, floor(x/y)=→"CurTime":sgl)
                              n236 = feedback #1(sgl 0.0) -> (w512:sgl)
                              n237 = feedback-in #1(w497) -> ()
                              n238 = Build Array (concatenate)(w512, w498) -> (w496:sgl[])
                              n239 = Build Array (concatenate)(w498, w497) -> (w494:sgl[])
                              n240 = Equal?(x=w496, y=w495) -> (x = y?=w492:bool[])
                              n241 = Equal?(x=w495, y=w494) -> (x = y?=w491:bool[])
                              n242 = Boolean To (0,1)(Boolean=w491) -> (0, 1=w489:i16[])
                              n243 = Boolean To (0,1)(Boolean=w492) -> (0, 1=w490:i16[])
                              n244 = Less?(x=w490, y=w489) -> (x < y?=w493:bool[])
                              n245 = Boolean To (0,1)(Boolean=w493) -> (0, 1=w514:i16[])
                              n246 = Add Array Elements(numeric array=w514) -> (sum=w515:i16)
                              n247 = Add(x=w515, y=w501) -> (x+y=w506:u32)
                            }
                            frame #1 {
                              n248 = To Unsigned Word Integer(number=w544) -> (unsigned 16bit integer=w545:u16[])
                              n249 = for {
                                tunnel: w545 -> [w572] mode=indexing
                                tunnel: [w559] -> w527 mode=indexing
                                n250 = Number To Boolean Array(number=w572) -> (Boolean array=w571:bool[])
                                n251 = Index Array(array=w571, index #1=7, index #2=6, index #3=4, index #4=3, index #5=2, index #6=0) -> (element #1=w570:bool, element #2=w569:bool, element #3=w568:bool, element #4=w567:bool, element #5=w566:bool, element #6=w558:bool)
                                n252 = Build Array(w570, w569, w568, w567, w566, w558) -> (w560:bool[])
                                n253 = Boolean To (0,1)(Boolean=w560) -> (0, 1=w559:i16[])
                              }
                              n254 = Array Size(array=w544) -> (size(s)=w551:i32)
                              n255 = Negate(x=w551) -> (-x=w549:i32)
                              n256 = for {
                                N: 6 -> [_]
                                tunnel: w543 -> [w556]
                                tunnel: w549 -> [w553]
                                tunnel: [w552] -> w550 mode=indexing
                                i -> [w555]
                                n257 = Index Array(array=w556, index (col)=w555) -> (element=w554:u8[])  [unwired: 1 in]
                                n258 = Rotate 1D Array(1:w554, 2:w553) -> (0:w552:u8[])
                              }
                              n259 = Subtract(x=w535, y=w551) -> (x-y=w546:u32)
                              n260 = Transpose 2D Array(2D array=w550) -> (transposed array=w533:u8[][])
                              n261 = Array Size(array=w533) -> (size(s)=w534:i32[])
                              n262 = Replace Array Subset(array=w533, new element=w527, index (row)=w546, index (col)=0 ("disabled index (col)")) -> (w538:u8[][])
                              n263 = Index Array(array=w534) -> ()  [unwired: 1 in, 1 out]
                              n264 = Index Array(array=w527, index (col) #1=0, index (col) #2=1, index (col) #3=2, index (col) #4=3) -> (element #1=w528:i16[], element #2=w526:i16[], element #3=w525:i16[], element #4=w524:i16[])  [unwired: 4 in]
                              n265 = Bundle By Name ("Build Digital Data")("data"=w538) -> (w540:digitaldata)  [unwired: 1 in]
                              n266 = To Time Stamp(1:10.0 ("number")) -> (0:w542:timestamp)
                              n267 = Add Array Elements(numeric array=w528) -> (sum=w523:i16)
                              n268 = Add Array Elements(numeric array=w525) -> (sum=w522:i16)
                              n269 = Add Array Elements(numeric array=w526) -> (sum=w520:i16)
                              n270 = Add Array Elements(numeric array=w524) -> (sum=w521:i16)
                              n271 = call <vilib>:"DWDT Empty Digital.vi"() -> ("digital waveform out"=w539:digitalwaveform)  [unwired: 5 in]
                              n272 = Build Array(w523, w520, w522, w521) -> (w519:i16[])
                              n273 = Bundle By Name ("Build Waveform")(cluster=w539, "Y"=w540, "dt"=w536, "t0"=w542) -> (→"Digital Waveform Graph":digitalwaveform)
                              n274 = Add(x=w519, y=w518) -> (x+y=w517:u32[])
                            }
                          }
                        }
                        frame True {
                          n275 = local read "stop - local"() -> (w576:bool)
                        }
                      }
                      n276 = Index Array(array=w455, index #1=0, index #2=1, index #3=2, index #4=3) -> (element #1=w452:u32, element #2=w453:u32, element #3=w450:u32, element #4=w449:u32)
                      n277 = local write "reward#"(w461) -> ()
                      n278 = Add(x=w452, y=w453) -> (x+y=w454:u32)
                      n279 = Add(x=w450, y=w449) -> (x+y=w451:u32)
                      n280 = Divide(x=w452, y=w454) -> (x/y=w445:dbl)
                      n281 = Divide(x=w453, y=w454) -> (x/y=w446:dbl)
                      n282 = Divide(x=w450, y=w451) -> (x/y=w448:dbl)
                      n283 = Divide(x=w449, y=w451) -> (x/y=w447:dbl)
                      n284 = local write "rightReward"(w445) -> ()
                      n285 = local write "leftReward"(w446) -> ()
                      n286 = local write "rightLick"(w448) -> ()
                      n287 = local write "leftLick"(w447) -> ()
                      n288 = node-c288() -> ()  [unwired: 1 in, 1 out]
                    }
                    n289 = timed-loop {
                      timing: w334 -> [_]
                      timing-out: [_] -> w333
                      tunnel: w313 -> [w417]
                      tunnel: [w413] -> w332
                      shift-right: [w412] -> w331
                      shift-left: w314 -> [w416]
                      tunnel: w330 -> [w411]
                      tunnel: w329 -> [w410]
                      tunnel: [w409] -> w328
                      tunnel: [w408] -> w327
                      stop <- w407 stop-if-true
                      n290 = node-c288() -> ()  [unwired: 1 in, 1 out]
                      n291 = Dequeue Element(queue=w417, timeout in ms (-1)=0, error in (no error)=w416) -> (queue out=w413:refnum<queue>, element=w414:sgl[], timed out?=w415:bool, error out=w412:errorcluster)
                      n292 = case shown="False" w415 {
                        tunnel: w414 -> [w423 _]
                        tunnel: w411 -> [w422 w437]
                        tunnel: w410 -> [w421 w436]
                        tunnel: [w420 w437] -> w409
                        tunnel: [w419 w436] -> w408
                        tunnel: [_ w435] -> w407
                        frame False {
                          n293 = local read "Save data"() -> (w424:bool)
                          n294 = case shown="True" w424 {
                            tunnel: w422 -> [w425 w434]
                            tunnel: w421 -> [w426 w433]
                            tunnel: w423 -> [_ w428]
                            tunnel: [w426 w430] -> w419
                            tunnel: [w425 w429] -> w420
                            frame False {
                            }
                            frame True {
                              n295 = To Single Precision Float(number=w428) -> (single precision float=w427:sgl[])
                              n296 = Write to Binary File(file (use dialog)=w434, data=w427, error in=w433, 5:FALSE ("prepend array or string size? (T)"), 9:T3."little-endian" ("byte order (0:big-endian, network order)")) -> (refnum out=w429:refnum<file>, error out=w430:errorcluster)  [unwired: 1 in, 1 out]
                            }
                          }
                        }
                        frame True {
                          n297 = local read "stop - local"() -> (w435:bool)
                        }
                      }
                      n298 = node-c288() -> ()  [unwired: 1 in, 1 out]
                    }
                    n299 = timed-loop {
                      timing: w367 -> [_]
                      timing-out: [_] -> w366
                      tunnel: w317 -> [w1133]
                      tunnel: [w1151] -> w362
                      tunnel: w315 -> [w1150]
                      tunnel: w311 -> [w1149]
                      tunnel: w312 -> [w1148]
                      tunnel: w313 -> [w1147]
                      tunnel: w314 -> [w1146]
                      shift-right: [w1144] -> _
                      shift-left: w361 -> [w1145]
                      shift-right: [w1142] -> _
                      shift-left: w361 -> [w1143]
                      tunnel: [w1141] -> w319
                      tunnel: [w1140] -> w322
                      shift-right: [w1138] -> _
                      shift-left: u32 0 -> [w1139]
                      shift-right: [w1130] -> w359
                      shift-left: w316 -> [w1131]
                      stop <- w1127 stop-if-true
                      # "Ignore error stating the other\nendpoint has been destroyed."
                      n300 = node-c288() -> ()  [unwired: 1 in]
                      n301 = property class="Network Stream Endpoint"(reference=w1150, error in=w1131) -> (reference out=w1129:refnum<k21>, error out=w1134:errorcluster, "Connected"=w1154:bool, "AvailElmntsForRead"=w1155:i32)
                      n302 = local write "Available Elements for Writing"(w1155) -> ()
                      n303 = Not(x=w1154) -> (.not. x?=w1153:bool)
                      n304 = local write "Is Connected"(w1154) -> ()
                      n305 = shared-variable-read(w1129, w1134, w1133) -> (w1136:refnum<k21>, w1132:errorcluster, w1137:bool, w1135:sgl[])
                      n306 = Or(x=w1137, y=w1153) -> (x .or. y?=w1152:bool)
                      n307 = case shown="False" w1152 {
                        tunnel: w1136 -> [w1168 w1179]
                        tunnel: [w1168 w1179] -> w1151
                        tunnel: w1149 -> [w1172 _]
                        tunnel: w1148 -> [w1170 w1176]
                        tunnel: w1147 -> [w1171 _]
                        tunnel: w1146 -> [w1169 w1175]
                        tunnel: w1145 -> [w1166 w1178]
                        tunnel: [w1162 w1178] -> w1144
                        tunnel: w1143 -> [w1165 w1177]
                        tunnel: [w1164 w1177] -> w1142
                        tunnel: [w1161 w1176] -> w1141
                        tunnel: [w1160 w1175] -> w1140
                        tunnel: w1139 -> [w1159 w1174]
                        tunnel: [w1158 w1174] -> w1138
                        tunnel: w1135 -> [w1157 _]
                        tunnel: [w1156 w1173] -> w1128
                        tunnel: w1132 -> [w1156 w1173]
                        frame False {
                          n308 = Enqueue Element(queue=w1172, element=w1157, error in (no error)=w1170) -> (timed out?=w1167:bool, error out=w1161:errorcluster)  [unwired: 1 in, 1 out]
                          n309 = Enqueue Element(queue=w1171, element=w1157, error in (no error)=w1169) -> (timed out?=w1163:bool, error out=w1160:errorcluster)  [unwired: 1 in, 1 out]
                          n310 = Increment(x=w1159) -> (x+1=w1158:u32)
                          n311 = Or(x=w1167, y=w1166) -> (x .or. y?=w1162:bool)
                          n312 = Or(x=w1163, y=w1165) -> (x .or. y?=w1164:bool)
                          n313 = local write "stream counter"(w1158) -> ()
                          n314 = local write "saveTimeout"(w1164) -> ()
                          n315 = local write "dispTimeout"(w1162) -> ()
                        }
                        frame True {
                        }
                      }
                      n316 = shared-variable "Sabrina-RT1\\variables - network - RT (separate).lvlib\\stop - network"() -> (w1127:bool)  [unwired: 1 in, 1 out]
                      n317 = local write "stop - local"(w1127) -> ()
                      n318 = call "Remove_selected_error.vi"("error in (no error)"=w1128, "errorCode"=-314220) -> ("error out"=w1130:errorcluster)
                      n319 = node-c288() -> ()  [unwired: 1 in, 1 out]
                    }
                    n320 = timed-loop {
                      timing: w358 -> [_]
                      timing-out: [_] -> w357
                      tunnel: w356 -> [w618]
                      tunnel: w355 -> [w617]
                      shift-right: [w615] -> _
                      shift-left: w354 -> [w616]
                      tunnel: [w614] -> w353
                      tunnel: [w613] -> w352
                      shift-right: [w612] -> _
                      shift-left: 0 ("index") -> [w602]
                      shift-right: [w610] -> _
                      shift-left: FALSE -> [w611]
                      shift-right: [w608] -> w346
                      shift-left: w349 -> [w609]
                      tunnel: w282 -> [w606]
                      tunnel: w281 -> [w605]
                      tunnel: [w604] -> w296
                      tunnel: [w603] -> w295
                      shift-right: [w596] -> _
                      shift-left: w280 -> [w597]
                      stop <- w607 stop-if-true
                      n321 = node-c288() -> ()  [unwired: 1 in, 1 out]
                      n322 = local read "stateBusy"() -> (w621:bool)
                      n323 = local read "forceLeftTrial"() -> (w599:bool)
                      n324 = local read "forceRightTrial"() -> (w601:bool)
                      n325 = local read "VSbusy"() -> (w620:bool)
                      n326 = Exclusive Or(1:w601, 2:w599) -> (0:w600:bool)
                      n327 = case shown="True" w600 {
                        tunnel: w602 -> [_ w624]
                        tunnel: w599 -> [_ w626]
                        tunnel: [w622 w625] -> w598
                        tunnel: w597 -> [w622 w623]
                        frame False {
                        }
                        frame True {
                          n328 = Select(t=1 ("index"), s=w626, f=2 ("index")) -> (s? t:f=w629:i32)
                          n329 = Replace Array Subset(array=w623, new element=w629, index=w624) -> (w625:i32[])
                        }
                      }
                      n330 = Or(x=w621, y=w620) -> (x .or. y?=w619:bool)
                      n331 = case shown="False" w619 {
                        tunnel: w618 -> [w643 w925]
                        tunnel: w617 -> [w636 w924]
                        tunnel: w616 -> [w646 w923]
                        tunnel: [w635 w922] -> w615
                        tunnel: [w642 w921] -> w614
                        tunnel: [w637 w920] -> w613
                        tunnel: w602 -> [w633 w919]
                        tunnel: [w648 w918] -> w612
                        tunnel: w611 -> [w647 w915]
                        tunnel: [w634 w917] -> w610
                        tunnel: w609 -> [w645 w916]
                        tunnel: [w644 w916] -> w608
                        tunnel: [w632 w911] -> w604
                        tunnel: [w631 w912] -> w603
                        tunnel: w606 -> [w632 w914]
                        tunnel: w605 -> [w631 w913]
                        tunnel: w598 -> [w630 w910]
                        tunnel: [w630 w909] -> w596
                        frame False {
                          n332 = stacked-sequence {
                            seq-local: [_ w795 _] -> [_ _ w900]
                            tunnel: w633 -> [_ w790 w902]
                            tunnel: [_ _ w901] -> w648
                            tunnel: w647 -> [_ w834 _]
                            tunnel: w646 -> [_ w832 _]
                            tunnel: w645 -> [_ w792 _]
                            tunnel: [_ w826 _] -> w644
                            tunnel: [_ w824 _] -> w639
                            tunnel: [_ w800 _] -> w635
                            tunnel: [_ w795 _] -> w634
                            tunnel: w630 -> [_ w788 _]
                            frame #0 {
                              n333 = local read "No VS"() -> (w649:bool)
                              n334 = case shown="False" w649 {
                                frame True {
                                }
                                frame False {
                                n335 = local read "CurTrial#"() -> (w653:u16)
                                n336 = local read "autoTimeout"() -> (w657:bool)
                                n337 = case shown="True" w657 {
                                frame False {
                                }
                                frame True {
                                n338 = local read "curPerformance"() -> (w744:dbl)
                                n339 = local read "overallPerformance"() -> (w746:dbl)
                                n340 = local read "reward#"() -> (w747:i32)
                                n341 = Less?(x=w744, y=0.7) -> (x < y?=w749:bool)
                                n342 = Less?(x=w747, y=10 ("index")) -> (x < y?=w753:bool)
                                n343 = Less?(x=w746, y=0.3) -> (x < y?=w755:bool)
                                n344 = Or(x=w753, y=w755) -> (x .or. y?=w750:bool)
                                n345 = Not(x=w750) -> (.not. x?=w748:bool)
                                n346 = And(x=w748, y=w749) -> (x .and. y?=w751:bool)
                                n347 = case shown="True" w751 {
                                tunnel: [w759 w761] -> w752
                                frame False {
                                n348 = local read "timeout_uS"() -> (w759:u32)
                                }
                                frame True {
                                n349 = local read "CurTrial#"() -> (w760:u16)
                                n350 = Quotient & Remainder(x=w760, y="updateEveryTrial#") -> (x-y*floor(x/y)=w769:u16)  [unwired: 1 out]
                                n351 = Equal?(x=0.0, y=w769) -> (x = y?=w768:bool)
                                n352 = local read "timeout_uS"() -> (w765:u32)
                                n353 = Add(x=1000000, y=w765) -> (x+y=w766:u32)
                                n354 = Select(t=w766, s=w768, f=w765) -> (s? t:f=w763:u32)
                                n355 = Less?(x=w763, y="maxTimeout") -> (x < y?=w764:bool)
                                n356 = Select(t=w763, s=w764, f="maxTimeout") -> (s? t:f=w761:u32)
                                }
                                }
                                n357 = Select(t=0, s=w750, f=w752) -> (s? t:f=w757:u32)
                                n358 = local write "timeout_uS"(w757) -> ()
                                }
                                }
                                n359 = local read "reward#"() -> (w654:i32)
                                n360 = local read "autoCorrTrial"() -> (w658:bool)
                                n361 = Divide(x=w654, y=w653) -> (x/y=w652:dbl)
                                n362 = local write "overallPerformance"(w652) -> ()
                                n363 = case shown="True" w658 {
                                frame False {
                                }
                                frame True {
                                n364 = local read "overallPerformance"() -> (w772:dbl)
                                n365 = local read "rightReward"() -> (w781:dbl)
                                n366 = local read "leftReward"() -> (w773:dbl)
                                n367 = local read "reward#"() -> (w774:i32)
                                n368 = Greater Or Equal?(x=w774, y=10 ("index")) -> (x >= y?=w777:bool)
                                n369 = Max & Min(x=w781, y=w773) -> (max(x,y)=w785:dbl)  [unwired: 1 out]
                                n370 = Greater Or Equal?(x=w772, y=0.5) -> (x >= y?=w775:bool)
                                n371 = Less?(x=w785, y=0.55 ("number")) -> (x < y?=w778:bool)
                                n372 = And(x=w778, y=w775) -> (x .and. y?=w776:bool)
                                n373 = Select(t=FALSE, s=w776, f=w777) -> (s? t:f=w783:bool)
                                n374 = local write "forceCorrTrial"(w783) -> ()
                                }
                                }
                                n375 = local read "autoDelay"() -> (w651:bool)
                                n376 = case shown="True" w651 {
                                tunnel: [w670 w674] -> w655
                                frame False {
                                n377 = local read "overallPerformance"() -> (w670:dbl)
                                }
                                frame True {
                                n378 = local read "reward#"() -> (w671:i32)
                                n379 = Greater?(x=w671, y=u16 11) -> (0:w672:bool)
                                n380 = case shown="True" w672 {
                                tunnel: [w682 w693] -> w674
                                tunnel: w671 -> [w680 w686]
                                frame False {
                                n381 = Equal?(x=w680, y=u16 11) -> (x = y?=w679:bool)
                                n382 = local read "overallPerformance"() -> (w682:dbl)
                                n383 = local read "VS type"() -> (w677:string)
                                n384 = case shown="\"DelayedMatchToSampleMove\", Default" w677 {
                                tunnel: [w683 w685] -> w676
                                tunnel: [w683 u32 0 ("delay_uS")] -> w675
                                frame "DelayedMatchToSampleMove", Default {
                                n385 = local read "maxDelay"() -> (w683:i32)
                                }
                                frame "DelayedMatchToSample" {
                                n386 = local read "minDelay"() -> (w685:i32)
                                }
                                }
                                n387 = Select(t=w676, s=w679, f=w675) -> (s? t:f=w678:u32)
                                n388 = local write "delay_uS"(w678) -> ()
                                }
                                frame True {
                                n389 = local read "newStartReward#"() -> (w695:i32)
                                n390 = local read "newStartTrial#"() -> (w697:i32)
                                n391 = local read "contNoRewardAccum"() -> (w696:i32)
                                n392 = local read "CurTrial# (remote)"() -> (w687:u16)
                                n393 = Subtract(x=w686, y=w695) -> (x-y=w688:i32)
                                n394 = local read "contReward"() -> (w698:i32)
                                n395 = Subtract(x=w687, y=w697) -> (x-y=w691:i32)
                                n396 = Subtract(x=w691, y=w696) -> (x-y=w694:i32)
                                n397 = Less?(x=10 ("index"), y=w691) -> (x < y?=w690:bool)
                                n398 = Greater Or Equal?(x=w698, y=4) -> (x >= y?=w703:bool)
                                n399 = Divide(x=w688, y=w694) -> (x/y=w693:dbl)
                                n400 = Greater?(x=w686, y=14) -> (0:w702:bool)
                                n401 = And(x=w702, y=w703) -> (x .and. y?=w701:bool)
                                n402 = Greater?(x=w693, y=0.7 ("number")) -> (0:w689:bool)
                                n403 = Compound Arithmetic op=AND(w701, w690, w689) -> (w704:bool)
                                n404 = case shown="True" w704 {
                                tunnel: w687 -> [_ w712]
                                tunnel: w686 -> [_ w711]
                                frame False {
                                }
                                frame True {
                                w710 = 0
                                n405 = local read "delay_uS"() -> (w709:u32)
                                n406 = local write "newStartReward#"(w711) -> ()
                                n407 = local write "newStartTrial#"(w712) -> ()
                                n408 = local read "VS type"() -> (w707:string)
                                n409 = case shown="\"DelayedMatchToSample\"" w707 {
                                tunnel: w709 -> [w717 w722]
                                tunnel: 200000.0 ("number") -> [w716 w721]
                                tunnel: [w713 w719] -> w708
                                frame "DelayedMatchToSampleMove", Default {
                                n410 = Subtract(x=w717, y=w716) -> (x-y=w715:dbl)
                                n411 = local read "minDelay"() -> (w714:i32)
                                n412 = Max & Min(x=w714, y=w715) -> (max(x,y)=w713:dbl)  [unwired: 1 out]
                                }
                                frame "DelayedMatchToSample" {
                                n413 = Add(x=w722, y=w721) -> (x+y=w720:dbl)
                                n414 = local read "maxDelay"() -> (w718:i32)
                                n415 = Max & Min(x=w718, y=w720) -> (min(x,y)=w719:dbl)  [unwired: 1 out]
                                }
                                }
                                n416 = local write "contNoRewardAccum"(w710) -> ()
                                n417 = local write "contReward"(w710) -> ()
                                n418 = local write "delay_uS"(w708) -> ()
                                }
                                }
                                }
                                }
                                }
                                }
                                n419 = local read "autoAllowCorrection"() -> (w650:bool)
                                n420 = local write "curPerformance"(w655) -> ()
                                n421 = local read "autoStop"() -> (w656:bool)
                                n422 = case shown="True" w656 {
                                frame False {
                                }
                                frame True {
                                n423 = local read "overallPerformance"() -> (w738:dbl)
                                n424 = Multiply(x=0.9 ("y"), y="autoStopAtReward#") -> (x*y=w732:dbl)
                                n425 = Less?(x=w738, y=0.7) -> (x < y?=w735:bool)
                                n426 = local read "waterPunish"() -> (w736:bool)
                                n427 = And(x=w735, y=w736) -> (x .and. y?=w737:bool)
                                n428 = Select(t=w732, s=w737, f="autoStopAtReward#") -> (s? t:f=w739:dbl)
                                n429 = local read "contNoReward"() -> (w725:i32)
                                n430 = local read "reward#"() -> (w730:i32)
                                n431 = Greater Or Equal?(x=w730, y=w739) -> (x >= y?=w742:bool)
                                n432 = Greater Or Equal?(x=w725, y=30 ("index")) -> (x >= y?=w728:bool)
                                n433 = Greater Or Equal?(x=w730, y=180 ("index")) -> (x >= y?=w727:bool)
                                n434 = Greater Or Equal?(x=w725, y=50 ("index")) -> (x >= y?=w726:bool)
                                n435 = And(x=w728, y=w727) -> (x .and. y?=w723:bool)
                                n436 = Compound Arithmetic op=OR(w742, w726, w723) -> (w741:bool)
                                n437 = case shown="True" w741 {
                                frame False {
                                }
                                frame True {
                                n438 = local write "run-stop"(FALSE) -> ()
                                }
                                }
                                }
                                }
                                n439 = case shown="True" w650 {
                                frame False {
                                }
                                frame True {
                                n440 = local read "contNoReward"() -> (w662:i32)
                                n441 = Greater?(x=w662, y=3 ("index")) -> (0:w659:bool)
                                n442 = case shown="False" w659 {
                                tunnel: [w663 TRUE] -> w660
                                frame False {
                                n443 = local read "reward#"() -> (w668:i32)
                                n444 = Greater Or Equal?(x=w668, y=10 ("index")) -> (x >= y?=w666:bool)
                                n445 = Select(t=FALSE, s=w666, f=TRUE) -> (s? t:f=w663:bool)
                                }
                                frame True {
                                }
                                }
                                n446 = local write "allowCorrection"(w660) -> ()
                                }
                                }
                                }
                              }
                            }
                            frame #1 {
                              # "beh para (20)"
                              n447 = local read "delay_uS"() -> (w822:u32)
                              n448 = local read "rewardPeriod_uS"() -> (w821:u32)
                              n449 = local read "rwdrefPeriod_uS"() -> (w820:u32)
                              n450 = local read "waterOn_uS"() -> (w819:u32)
                              n451 = local read "shockOn_uS"() -> (w818:u32)
                              n452 = local read "timeout_uS"() -> (w817:u32)
                              n453 = local read "lickReward"() -> (w816:bool)
                              n454 = local read "toneReward"() -> (w815:bool)
                              n455 = local read "allowPunish"() -> (w814:bool)
                              n456 = local read "manualShock"() -> (w813:bool)
                              n457 = local read "manualWaterLeft"() -> (w812:bool)
                              n458 = local read "manualWaterRight"() -> (w811:bool)
                              n459 = local read "lickThreshold_V"() -> (w810:fxp<+/-,16,5>)
                              n460 = local read "vsThreshold_V"() -> (w809:fxp<+/-,16,5>)
                              n461 = local read "audioThreshold_V"() -> (w808:fxp<+/-,16,5>)
                              n462 = local read "audioOffState_V"() -> (w805:fxp<+/-,16,5>)
                              n463 = local read "audioFilterPeriod_uS"() -> (w807:i32)
                              n464 = local read "vsFilterPeriod_uS"() -> (w806:i32)
                              n465 = local read "allowCorrection"() -> (w786:bool)
                              n466 = Index Array(array=w788, index=w790) -> (element=w791:i32)
                              n467 = Build Array(w822, w821, w820, w819, w818, w817) -> (w804:u32[])
                              n468 = Build Array(w816, w815, w814, w813, w812, w811, w786) -> (w797:bool[])
                              n469 = Boolean To (0,1)(Boolean=w797) -> (0, 1=w796:i16[])
                              n470 = Build Array(w810, w809, w808, w805, w807, w806) -> (w803:fxp<+/-,43,32>[])
                              n471 = Initialize Array(sgl 0.0, 1) -> (w787:sgl[])
                              n472 = Build Array (concatenate)(w804, w796, w803, w791, w787) -> (w800:sgl[])
                              n473 = Array Size(array=w800) -> (size(s)=w799:i32)
                              n474 = Subtract(x=w800, y=w832) -> (x-y=w831:sgl[])
                              n475 = Reshape Array(w800, w799, 1 ("dimension size")) -> (w827:sgl[][])
                              n476 = Absolute Value(x=w831) -> (abs(x)=w829:sgl[])
                              n477 = Less?(x=w829, y=1e-06) -> (x < y?=w828:bool[])
                              n478 = Replace Array Subset(array=w792, new element=w827, index (row)=0 ("dimension size"), index (col)=w790) -> (w826:sgl[][])
                              n479 = for {
                                N: 19 ("dimension size") -> [_]
                                tunnel: w828 -> [w871] mode=indexing
                                tunnel: w800 -> [w870] mode=indexing
                                shift-right: [w867] -> w825
                                shift-left: "" -> [w868]
                                i -> [w869]
                                n480 = case shown="False" w871 {
                                tunnel: w870 -> [_ w880]
                                tunnel: w869 -> [_ w874]
                                tunnel: w868 -> [w872 w878]
                                tunnel: [w872 w877] -> w867
                                frame True {
                                }
                                frame False {
                                n481 = case shown="12" w874 {
                                tunnel: ["dly" "rwp" "rwf" "wdr" "shd" "tod" "lkr" "tlr" "alp" "msh" "mwl" "mwr" "alc" "lth" "vth" "ath" "aof" "afp" _ _ _] -> w873
                                frame 0, Default {
                                }
                                frame 1 {
                                }
                                frame 2 {
                                }
                                frame 3 {
                                }
                                frame 4 {
                                }
                                frame 5 {
                                }
                                frame 6 {
                                }
                                frame 7 {
                                }
                                frame 8 {
                                }
                                frame 9 {
                                }
                                frame 10 {
                                }
                                frame 11 {
                                }
                                frame 12 {
                                }
                                frame 13 {
                                }
                                frame 14 {
                                }
                                frame 15 {
                                }
                                frame 16 {
                                }
                                frame 17 {
                                }
                                frame 18 {
                                (unwired) "vfp"
                                }
                                frame 19 {
                                }
                                frame 20 {
                                }
                                }
                                n482 = Format Value(format string="%.3f", value (0)=w880) -> (output string=w875:string)  [unwired: 1 in]
                                n483 = call <vilib>:"Space Constant.vi"() -> ("String"=w876:string)
                                n484 = Concatenate Strings(w878, w873, w876, w875, w876) -> (w877:string)
                                }
                                }
                              }
                              n485 = local read "VSmissed"() -> (w837:bool)
                              n486 = local read "stateMissed"() -> (w836:bool)
                              n487 = local read "CurTrial#"() -> (w840:u16)
                              n488 = local read "totalTrial#"() -> (w839:u16)
                              n489 = local read "run-stop"() -> (w835:bool)
                              n490 = Equal?(x=w840, y=w839) -> (x = y?=w838:bool)
                              n491 = Not(x=w835) -> (.not. x?=w833:bool)
                              n492 = Compound Arithmetic op=OR(w837, w836, w838) -> (w823:bool)
                              n493 = case shown="True" w823 {
                                frame False {
                                }
                                frame True {
                                n494 = local write "run-stop"(FALSE ("run-stop")) -> ()
                                }
                              }
                              n495 = Compound Arithmetic op=OR(w823, w833, w834) -> (w795:bool)
                              n496 = case shown="False" w795 {
                                tunnel: w825 -> [w844 _]
                                tunnel: [w843 w863] -> w824
                                tunnel: w791 -> [w841 _]
                                frame False {
                                n497 = flat-sequence {
                                tunnel: w844 -> [w845]
                                tunnel: [w845] -> w842
                                tunnel: [w859] -> w843
                                tunnel: w842 -> [w862]
                                tunnel: w841 -> [w856]
                                frame #0 {
                                n498 = disable-structure shown="Enabled" {
                                frame Disabled {
                                n499 = Random Number (0-1)() -> (number: 0 to 1=w848:dbl)
                                n500 = Multiply(x=w848, y=3000.0) -> (x*y=w850:dbl)
                                n501 = local read "ITI_ms"() -> (w846:dbl)
                                n502 = Add(x=w846, y=w850) -> (x+y=w849:dbl)
                                n503 = Wait (ms)(milliseconds to wait=w849) -> ()  [unwired: 1 out]
                                }
                                frame Enabled {
                                n504 = Random Number (0-1)() -> (number: 0 to 1=w853:dbl)
                                n505 = local read "ITI_ms"() -> (w851:dbl)
                                n506 = Multiply(x=w853, y=0) -> (x*y=w852:dbl)
                                n507 = Add(x=w851, y=w852) -> (x+y=w854:dbl)
                                n508 = Wait (ms)(milliseconds to wait=w854) -> ()  [unwired: 1 out]
                                }
                                }
                                }
                                frame #1 {
                                n509 = call <vilib>:"Space Constant.vi"() -> ("String"=w860:string)
                                n510 = Format Value(format string="%.3f", value (0)=w856) -> (output string=w857:string)  [unwired: 1 in]
                                n511 = Concatenate Strings(w862, "start" ("string"), w860, w857, w860) -> (w859:string)
                                }
                                }
                                }
                                frame True {
                                n512 = call <vilib>:"Space Constant.vi"() -> ("String"=w865:string)
                                n513 = Concatenate Strings("stop" ("string"), w865, "1.000" ("string"), w865) -> (w863:string)
                                n514 = call "generateTone.vi"() -> ()  [unwired: 12 in]
                                }
                              }
                            }
                            frame #2 {
                              n515 = case shown="False" w900 {
                                tunnel: w902 -> [w903 w908]
                                tunnel: [w903 w907] -> w901
                                frame True {
                                }
                                frame False {
                                n516 = Increment(x=w908) -> (x+1=w907:i32)
                                n517 = local read "No VS"() -> (w904:bool)
                                n518 = Not(x=w904) -> (.not. x?=w905:bool)
                                n519 = local write "CurTrial#"(w907) -> ()
                                n520 = local write "stateBusy"(TRUE) -> ()
                                n521 = local write "VSbusy"(w905) -> ()
                                }
                              }
                            }
                          }
                          n522 = local write "INFO"(w639) -> ()
                          n523 = local read "IP_broadcast"() -> (w640:string)
                          n524 = local read "port_remote"() -> (w638:u16)
                          n525 = String To IP(1:w640) -> (0:w641:u32)
                          n526 = UDP Write(address=w641, port or service name=w638, connection ID=w643, data in=w639, 8:w636) -> (error out=w637:errorcluster, 3:w642:refnum<k16>)  [unwired: 1 in]
                        }
                        frame True {
                          n527 = stacked-sequence {
                            tunnel: w925 -> [w979 _]
                            tunnel: w924 -> [w978 _]
                            tunnel: w923 -> [w974 _]
                            tunnel: [w937 _] -> w922
                            tunnel: [w932 _] -> w921
                            tunnel: [w933 _] -> w920
                            tunnel: w919 -> [w930 w1032]
                            tunnel: [_ w1031] -> w918
                            tunnel: [w960 _] -> w917
                            tunnel: w915 -> [w934 _]
                            tunnel: w914 -> [_ w1030]
                            tunnel: w913 -> [_ w1029]
                            tunnel: [_ w1028] -> w911
                            tunnel: [_ w1027] -> w912
                            tunnel: w910 -> [w927 w1025]
                            tunnel: [_ w1024] -> w909
                            frame #0 {
                              # "triakKey is not used here, may be deleted"
                              # "beh para (21)"
                              n528 = local read "delay_uS"() -> (w959:u32)
                              n529 = local read "rewardPeriod_uS"() -> (w958:u32)
                              n530 = local read "rwdrefPeriod_uS"() -> (w957:u32)
                              n531 = local read "waterOn_uS"() -> (w956:u32)
                              n532 = local read "shockOn_uS"() -> (w955:u32)
                              n533 = local read "timeout_uS"() -> (w954:u32)
                              n534 = local read "lickReward"() -> (w953:bool)
                              n535 = local read "toneReward"() -> (w952:bool)
                              n536 = local read "allowPunish"() -> (w951:bool)
                              n537 = local read "manualShock"() -> (w950:bool)
                              n538 = local read "manualWaterLeft"() -> (w949:bool)
                              n539 = local read "manualWaterRight"() -> (w948:bool)
                              n540 = local read "lickThreshold_V"() -> (w947:fxp<+/-,16,5>)
                              n541 = local read "vsThreshold_V"() -> (w946:fxp<+/-,16,5>)
                              n542 = local read "audioThreshold_V"() -> (w945:fxp<+/-,16,5>)
                              n543 = local read "audioOffState_V"() -> (w942:fxp<+/-,16,5>)
                              n544 = local read "audioFilterPeriod_uS"() -> (w944:i32)
                              n545 = local read "vsFilterPeriod_uS"() -> (w943:i32)
                              n546 = local read "allowCorrection"() -> (w926:bool)
                              n547 = Index Array(array=w927, index=w930) -> (element=w929:i32)
                              n548 = Build Array(w959, w958, w957, w956, w955, w954) -> (w941:u32[])
                              n549 = Build Array(w953, w952, w951, w950, w949, w948, w926) -> (w936:bool[])
                              n550 = Boolean To (0,1)(Boolean=w936) -> (0, 1=w935:i16[])
                              n551 = Build Array(w947, w946, w945, w942, w944, w943) -> (w940:fxp<+/-,43,32>[])
                              n552 = Initialize Array(sgl 0.0, 1) -> (w931:sgl[])
                              n553 = Build Array (concatenate)(w941, w935, w940, w929, w931) -> (w937:sgl[])
                              n554 = Subtract(x=w937, y=w974) -> (x-y=w977:sgl[])
                              n555 = Absolute Value(x=w977) -> (abs(x)=w976:sgl[])
                              n556 = Less?(x=w976, y=1e-06) -> (x < y?=w973:bool[])
                              n557 = for {
                                N: 19 ("dimension size") -> [_]
                                tunnel: w973 -> [w982] mode=indexing
                                shift-right: [w983] -> w969
                                shift-left: "" -> [w984]
                                tunnel: w937 -> [w981] mode=indexing
                                i -> [w985]
                                n558 = case shown="False" w982 {
                                tunnel: w985 -> [w993 _]
                                tunnel: w984 -> [w989 w1013]
                                tunnel: [w987 w1013] -> w983
                                tunnel: w981 -> [w986 _]
                                frame False {
                                n559 = case shown="15" w993 {
                                tunnel: ["dly" "rwp" "rwf" "wdr" "shd" "tod" "lkr" "tlr" "alp" "msh" "mwl" "mwr" "alc" "lth" "vth" "ath" "aof" "afp" "vfp" _ _] -> w988
                                frame 0, Default {
                                }
                                frame 1 {
                                }
                                frame 2 {
                                }
                                frame 3 {
                                }
                                frame 4 {
                                }
                                frame 5 {
                                }
                                frame 6 {
                                }
                                frame 7 {
                                }
                                frame 8 {
                                }
                                frame 9 {
                                }
                                frame 10 {
                                }
                                frame 11 {
                                }
                                frame 12 {
                                }
                                frame 13 {
                                }
                                frame 14 {
                                }
                                frame 15 {
                                }
                                frame 16 {
                                }
                                frame 17 {
                                }
                                frame 18 {
                                }
                                frame 19 {
                                }
                                frame 20 {
                                }
                                }
                                n560 = Format Value(format string="%.3f", value (0)=w986) -> (output string=w990:string)  [unwired: 1 in]
                                n561 = call <vilib>:"Space Constant.vi"() -> ("String"=w991:string)
                                n562 = Concatenate Strings(w989, w988, w991, w990, w991) -> (w987:string)
                                }
                                frame True {
                                }
                                }
                              }
                              n563 = String Length(string=w969) -> (length=w970:i32)
                              n564 = Not Equal To 0?(x=w970) -> (x != 0?=w971:bool)
                              n565 = case shown="True" w971 {
                                tunnel: w979 -> [w1014 w1023]
                                tunnel: w978 -> [w1015 w1022]
                                tunnel: w969 -> [_ w1018]
                                tunnel: [w1014 w1017] -> w932
                                tunnel: [w1015 w1016] -> w933
                                frame False {
                                }
                                frame True {
                                n566 = local read "IP_broadcast"() -> (w1020:string)
                                n567 = local read "port_remote"() -> (w1019:u16)
                                n568 = String To IP(1:w1020) -> (0:w1021:u32)
                                n569 = UDP Write(address=w1021, port or service name=w1019, connection ID=w1023, data in=w1018, 8:w1022) -> (error out=w1016:errorcluster, 3:w1017:refnum<k16>)  [unwired: 1 in]
                                }
                              }
                              n570 = local read "VSmissed"() -> (w964:bool)
                              n571 = local read "stateMissed"() -> (w965:bool)
                              n572 = local read "CurTrial#"() -> (w961:u16)
                              n573 = local read "totalTrial#"() -> (w962:u16)
                              n574 = local read "run-stop"() -> (w968:bool)
                              n575 = Equal?(x=w961, y=w962) -> (x = y?=w963:bool)
                              n576 = Not(x=w968) -> (.not. x?=w967:bool)
                              n577 = Compound Arithmetic op=OR(w964, w965, w963) -> (w966:bool)
                              n578 = case shown="False" w966 {
                                frame False {
                                }
                                frame True {
                                n579 = local write "run-stop"(FALSE ("run-stop")) -> ()
                                }
                              }
                              n580 = Compound Arithmetic op=OR(w966, w967, w934) -> (w960:bool)
                            }
                            frame #1 {
                              n581 = UDP Read(connection ID=w1030, timeout ms (25000)=0, 8:w1029) -> (data out=w1033:string, error out=w1038:errorcluster, 3:w1028:refnum<k16>, 6:w1034:u32)  [unwired: 1 in, 1 out]
                              n582 = String Length(string=w1033) -> (length=w1036:i32)
                              n583 = local write "Incoming data"(w1033) -> ()
                              n584 = Not Equal To 0?(x=w1036) -> (x != 0?=w1035:bool)
                              n585 = case shown="True" w1035 {
                                tunnel: w1034 -> [_ w1046]
                                tunnel: w1033 -> [_ w1052]
                                tunnel: w1032 -> [w1040 w1045]
                                tunnel: [w1040 w1043] -> w1031
                                tunnel: w1025 -> [w1039 w1042]
                                tunnel: [w1039 w1041] -> w1024
                                frame False {
                                }
                                frame True {
                                n586 = Scan From String(format string="%s %f ", input string=w1052, initial scan location=u32 0, default 1="no" ("default value 1"), default 2=-1.0 ("default value 2")) -> (output 1=w1047:string, output 2=w1044:dbl)  [unwired: 1 in, 3 out]
                                n587 = case shown="\"TrlDone\", Default" w1047 {
                                tunnel: w1046 -> [w1062]
                                tunnel: w1045 -> [w1055]
                                tunnel: w1044 -> [w1056]
                                tunnel: [w1055] -> w1043
                                tunnel: w1042 -> [w1054]
                                tunnel: [w1053] -> w1041
                                frame "TrlDone", Default {
                                n588 = local read "IP_RT"() -> (w1060:string)
                                n589 = IP To String(1:TRUE ("dot notation? (F)"), 2:w1062) -> (0:w1057:string)
                                n590 = Match True/False String(2:"" ("false string"), 3:w1060, 4:w1057) -> (0:w1058:bool)  [unwired: 1 out]
                                n591 = local write "Originating IP"(w1057) -> ()
                                n592 = case shown="True" w1058 {
                                tunnel: w1057 -> [w1069 _]
                                tunnel: w1055 -> [w1066 w1087]
                                tunnel: w1056 -> [w1065 w1081]
                                tunnel: w1054 -> [w1063 w1086]
                                tunnel: [w1063 w1085] -> w1053
                                frame False {
                                n593 = local read "IP_VS"() -> (w1068:string)
                                n594 = Match True/False String(2:"" ("false string"), 3:w1068, 4:w1069) -> (0:w1064:bool)  [unwired: 1 out]
                                n595 = case shown="True" w1064 {
                                tunnel: w1066 -> [_ w1076]
                                tunnel: w1065 -> [_ w1075]
                                frame False {
                                n596 = local write "Error 2"("Unknown source Error") -> ()
                                }
                                frame True {
                                n597 = Subtract(x=w1075, y=w1076) -> (x-y=w1074:dbl)
                                n598 = Absolute Value(x=w1074) -> (abs(x)=w1073:dbl)
                                n599 = local write "VSbusy"(FALSE) -> ()
                                n600 = Greater?(x=w1073, y=1e-06) -> (0:w1071:bool)
                                n601 = local write "VSmissed"(w1071) -> ()
                                }
                                }
                                }
                                frame True {
                                n602 = To Word Integer(number=w1081) -> (16bit integer=w1084:i16)
                                n603 = local read "forceCorrTrial"() -> (w1083:bool)
                                n604 = To Word Integer(number=w1081) -> (16bit integer=w1080:i16)
                                n605 = disable-structure shown="Disabled" {
                                disable-tunnel: w1081 -> [w1119 _]
                                disable-tunnel: w1087 -> [w1118 _]
                                frame Disabled {
                                n606 = Subtract(x=w1119, y=w1118) -> (x-y=w1117:dbl)
                                n607 = Absolute Value(x=w1117) -> (abs(x)=w1116:dbl)
                                n608 = Greater?(x=w1116, y=1e-06) -> (0:w1114:bool)
                                n609 = local write "stateMissed"(w1114) -> ()
                                }
                                frame Enabled {
                                }
                                }
                                n610 = local write "stateBusy"(FALSE) -> ()
                                n611 = case shown="1" w1080 {
                                tunnel: [w1091 0] -> w1082
                                tunnel: [0 w1101] -> w1079
                                tunnel: [w1089 w1093] -> w1078
                                frame 0, Default {
                                n612 = local read "contNoRewardAccum"() -> (w1089:i32)
                                n613 = local read "contNoReward"() -> (w1092:i32)
                                n614 = Increment(x=w1092) -> (x+1=w1091:i32)
                                }
                                frame 1 {
                                n615 = local read "contNoReward"() -> (w1097:i32)
                                n616 = Greater?(x=w1097, y=5) -> (0:w1098:bool)
                                n617 = Select(t=w1097, s=w1098, f=0) -> (s? t:f=w1096:i32)
                                n618 = local read "contNoRewardAccum"() -> (w1095:i32)
                                n619 = local read "contReward"() -> (w1100:i32)
                                n620 = Add(x=w1096, y=w1095) -> (x+y=w1093:i32)
                                n621 = Increment(x=w1100) -> (x+1=w1101:i32)
                                }
                                }
                                n622 = case shown="True" w1083 {
                                tunnel: w1087 -> [_ w1107]
                                tunnel: w1086 -> [w1103 w1106]
                                tunnel: [w1103 w1105] -> w1085
                                tunnel: w1084 -> [_ w1104]
                                frame False {
                                }
                                frame True {
                                n623 = case shown="0" w1104 {
                                tunnel: w1107 -> [w1110 _]
                                tunnel: w1106 -> [w1112 w1113]
                                tunnel: [w1111 w1113] -> w1105
                                frame 0 {
                                n624 = Decrement(x=w1110) -> (x-1=w1109:i32)
                                n625 = Index Array(array=w1112, index=w1109) -> ()  [unwired: 1 out]
                                n626 = Replace Array Subset(array=w1112, new element=0, index=w1110) -> (w1111:i32[])
                                }
                                frame 1, Default {
                                }
                                }
                                }
                                }
                                n627 = local write "contNoReward"(w1082) -> ()
                                n628 = local write "contReward"(w1079) -> ()
                                n629 = local write "contNoRewardAccum"(w1078) -> ()
                                }
                                }
                                }
                                }
                                }
                              }
                              n630 = call "Remove_selected_error.vi"("error in (no error)"=w1038, "errorCode"=56) -> ("error out"=w1027:errorcluster)
                            }
                          }
                        }
                      }
                      n631 = local read "stop - local"() -> (w607:bool)
                      n632 = node-c288() -> ()  [unwired: 1 in, 1 out]
                    }
                    n633 = node-c288(w333) -> ()  [unwired: 1 out]
                    n634 = Release Queue(queue=w332, error in (no error)=w331) -> (error out=w321:errorcluster)  [unwired: 1 in, 2 out]
                    n635 = To Single Precision Float(number=w346) -> (single precision float=w348:sgl[][])
                    n636 = local read "Save data"() -> (w347:bool)
                    n637 = node-c288(w366) -> ()  [unwired: 1 out]
                    n638 = case shown="True" w347 {
                      tunnel: w327 -> [w581 w595]
                      tunnel: w328 -> [_ w594]
                      tunnel: w348 -> [_ w585]
                      tunnel: [w581 w582] -> w320
                      frame False {
                      }
                      frame True {
                        n639 = Multiply(x=502, y=4) -> (x*y=w590:i32)
                        n640 = Set File Position(offset (in bytes) (0)=w590, refnum=w594, from (0:start)=enum16{"start", "end", "current"}."start", error in=w595) -> (refnum out=w587:refnum<file>, error out=w588:errorcluster)
                        n641 = Write to Binary File(file (use dialog)=w587, data=w585, error in=w588, 5:FALSE ("prepend array or string size? (T)"), 9:T3."little-endian" ("byte order (0:big-endian, network order)")) -> (refnum out=w583:refnum<file>, error out=w584:errorcluster)  [unwired: 1 in, 1 out]
                        n642 = Close File(refnum=w583, error in=w584) -> (error out=w582:errorcluster)  [unwired: 1 out]
                      }
                    }
                    n643 = node-c288(w335) -> ()  [unwired: 1 out]
                    n644 = Release Queue(queue=w326, error in (no error)=w325) -> (error out=w300:errorcluster)  [unwired: 1 in, 2 out]
                    n645 = Destroy Stream Endpoint(8:w359, 11:w362) -> (0:w323:errorcluster)
                    n646 = node-c288(w357) -> ()  [unwired: 1 out]
                    n647 = flat-sequence {
                      tunnel: w318 -> [w405]
                      frame #0 {
                        n648 = call <vilib>:"Simple Error Handler.vi"("error in (no error)"=w405) -> ()  [unwired: 4 in, 5 out]
                        n649 = shared-variable "Sabrina-RT1\\variables - network - RT (separate).lvlib\\stop - network"(FALSE ("stop - network")) -> ()  [unwired: 1 in, 1 out]
                      }
                    }
                    n650 = UDP Close(connection ID=w296, 8:w295) -> ()  [unwired: 2 out]
                    n651 = UDP Close(connection ID=w353, 8:w352) -> (error out=w324:errorcluster)  [unwired: 1 out]
                    n652 = Merge Errors(w324, w323, w319, w322, w300, w321, w320) -> (w318:errorcluster)
                  }
                }
              }
              frame 2 {
                n653 = local read "IP_host"() -> (w1190:string)
                n654 = local read "port_local"() -> (w1191:u16)
                n655 = String To IP(1:w1190) -> (0:w1189:u32)
                n656 = UDP Open(7:w1189, 11:w1191) -> (port=w1193:refnum<k16>, 0:w1194:errorcluster)  [unwired: 3 in, 1 out]
                n657 = local read "IP_broadcast"() -> (w1187:string)
                n658 = local read "port_remote"() -> (w1188:u16)
                n659 = String To IP(1:w1187) -> (0:w1192:u32)
                n660 = UDP Write(address=w1192, port or service name=w1188, connection ID=w1193, data in="exit 1.000 ", 8:w1194) -> (error out=w1196:errorcluster, 3:w1195:refnum<k16>)  [unwired: 1 in]
                n661 = UDP Close(connection ID=w1195, 8:w1196) -> (error out=w1197:errorcluster)  [unwired: 1 out]
                n662 = call <vilib>:"Simple Error Handler.vi"("error in (no error)"=w1197) -> ()  [unwired: 4 in, 5 out]
              }
            }
          }
          frame #2 {
            n663 = Wait (ms)(milliseconds to wait=u32 5) -> ()  [unwired: 1 out]
          }
        }
      }
    }
  }
